vi "Experiment 21.vi"() -> ()   [LabVIEW 2026]
doc: "Experiment 21\nThis experiment is like Experiment 19 but uses while loops instead of for loops."
uses:
  <vilib>/AdvancedString/1D String Array to Delimited String (string).vi
  <vilib>/Analysis/baseanly.llb/Mean (DBL).vi
  <vilib>/Analysis/NI_AALBase.lvlib
panel:
  out "No. Of Iterations Executed - Loop 14":i32
  out "Output - Loop 14":dbl[](array[numeric]) format="%.3f"
  out "No. Of Iterations Executed - Loop 13":i32
  out "Output - Loop 13":dbl[](array[numeric]) format="%.3f"
  out "No. Of Iterations Executed - Loop 12":i32
  out "Output - Loop 12":dbl[](array[numeric]) format="%.3f"
  out "No. Of Iterations Executed - Loop 11":i32
  out "Output - Loop 11":dbl[](array[numeric]) format="%.3f"
  out "No. Of Iterations As Block Of Text (easy to copy into Excel)":string
  out "No. Of Iterations Executed - Loop 10":i32
  out "Output - Loop 10":dbl[](array[numeric]) format="%.3f"
  out "No. Of Iterations Executed - Loop 9":i32
  out "Output - Loop 9":dbl[](array[numeric]) format="%.3f"
  out "No. Of Iterations Executed - Loop 8":i32
  out "Output - Loop 8":dbl[](array[numeric]) format="%.3f"
  out "No. Of Iterations Executed - Loop 7":i32
  out "Output - Loop 7":dbl[](array[numeric]) format="%.3f"
  out "No. Of Iterations Executed - Loop 6":i32
  out "Output - Loop 6":dbl[](array[numeric]) format="%.3f"
  out "No. Of Iterations Executed - Loop 5":i32
  out "Output - Loop 5":dbl[](array[numeric]) format="%.3f"
  out "No. Of Iterations Executed - Loop 4":i32
  out "Output - Loop 4":dbl[](array[numeric]) format="%.3f"
  out "No. Of Iterations Executed - Loop 3":i32
  out "Output - Loop 3":dbl[](array[numeric]) format="%.3f"
  out "Avg. No. Of Iterations Executed - All Loops":dbl format="%.1f"
  out "No. Of Iterations Executed - Loop 2":i32
  out "Output - Loop 2":dbl[](array[numeric]) format="%.3f"
  out "No. Of Iterations Executed - Loop 1":i32
  out "Output - Loop 1":dbl[](array[numeric]) format="%.3f"
  out "Stop VI?":bool
  # "Experiment 21"
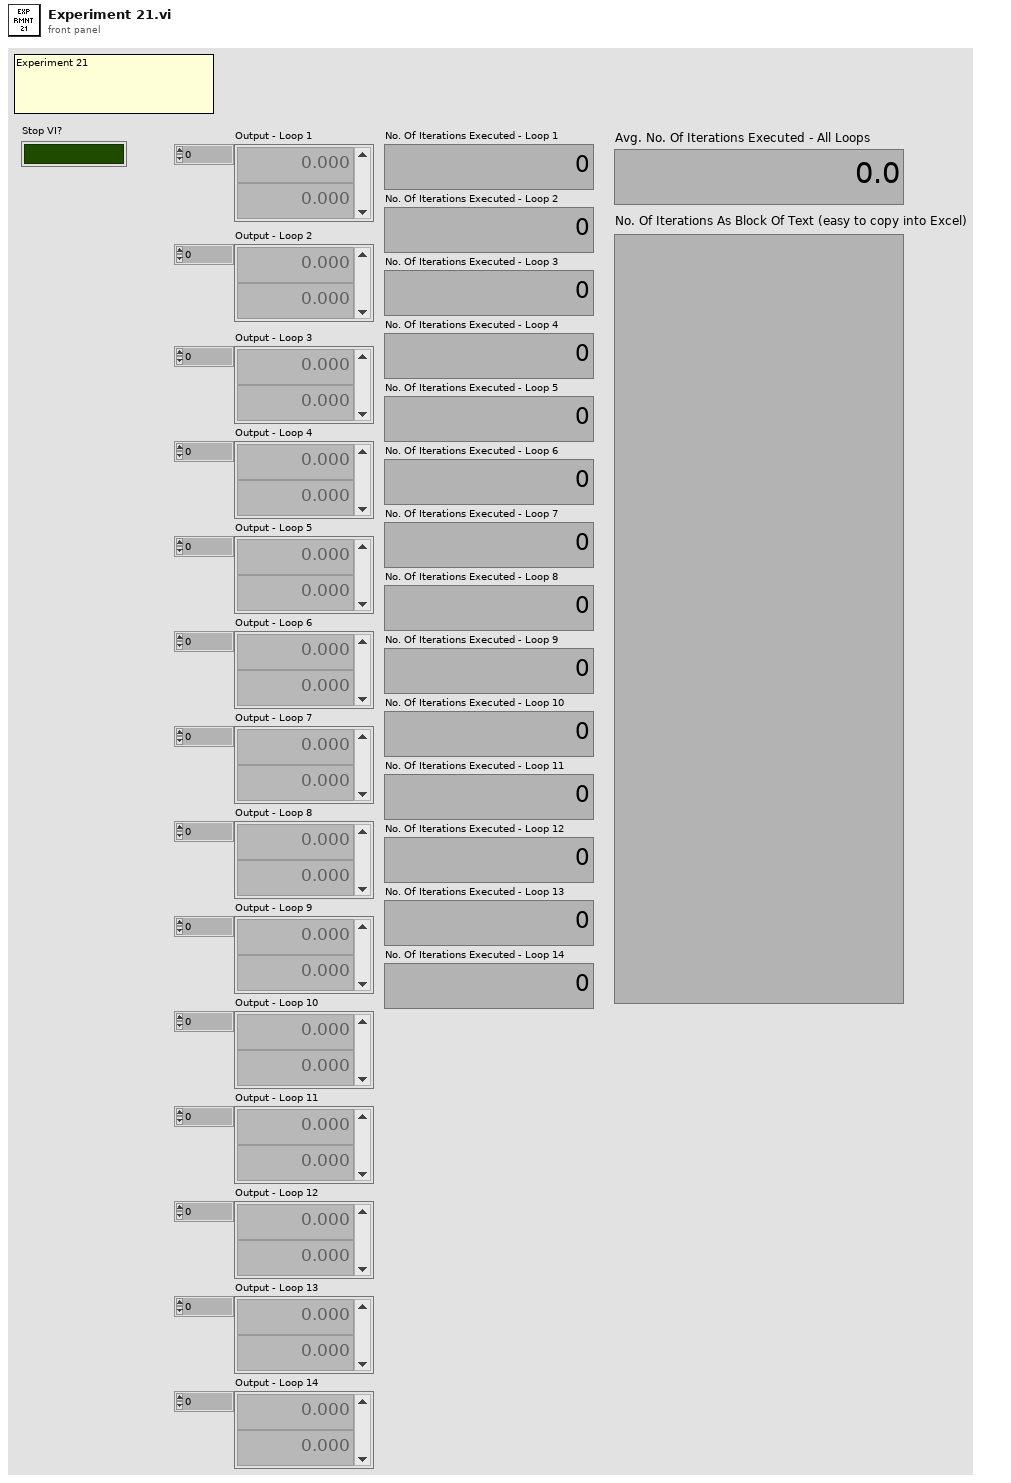
[diagram p1: front panel]
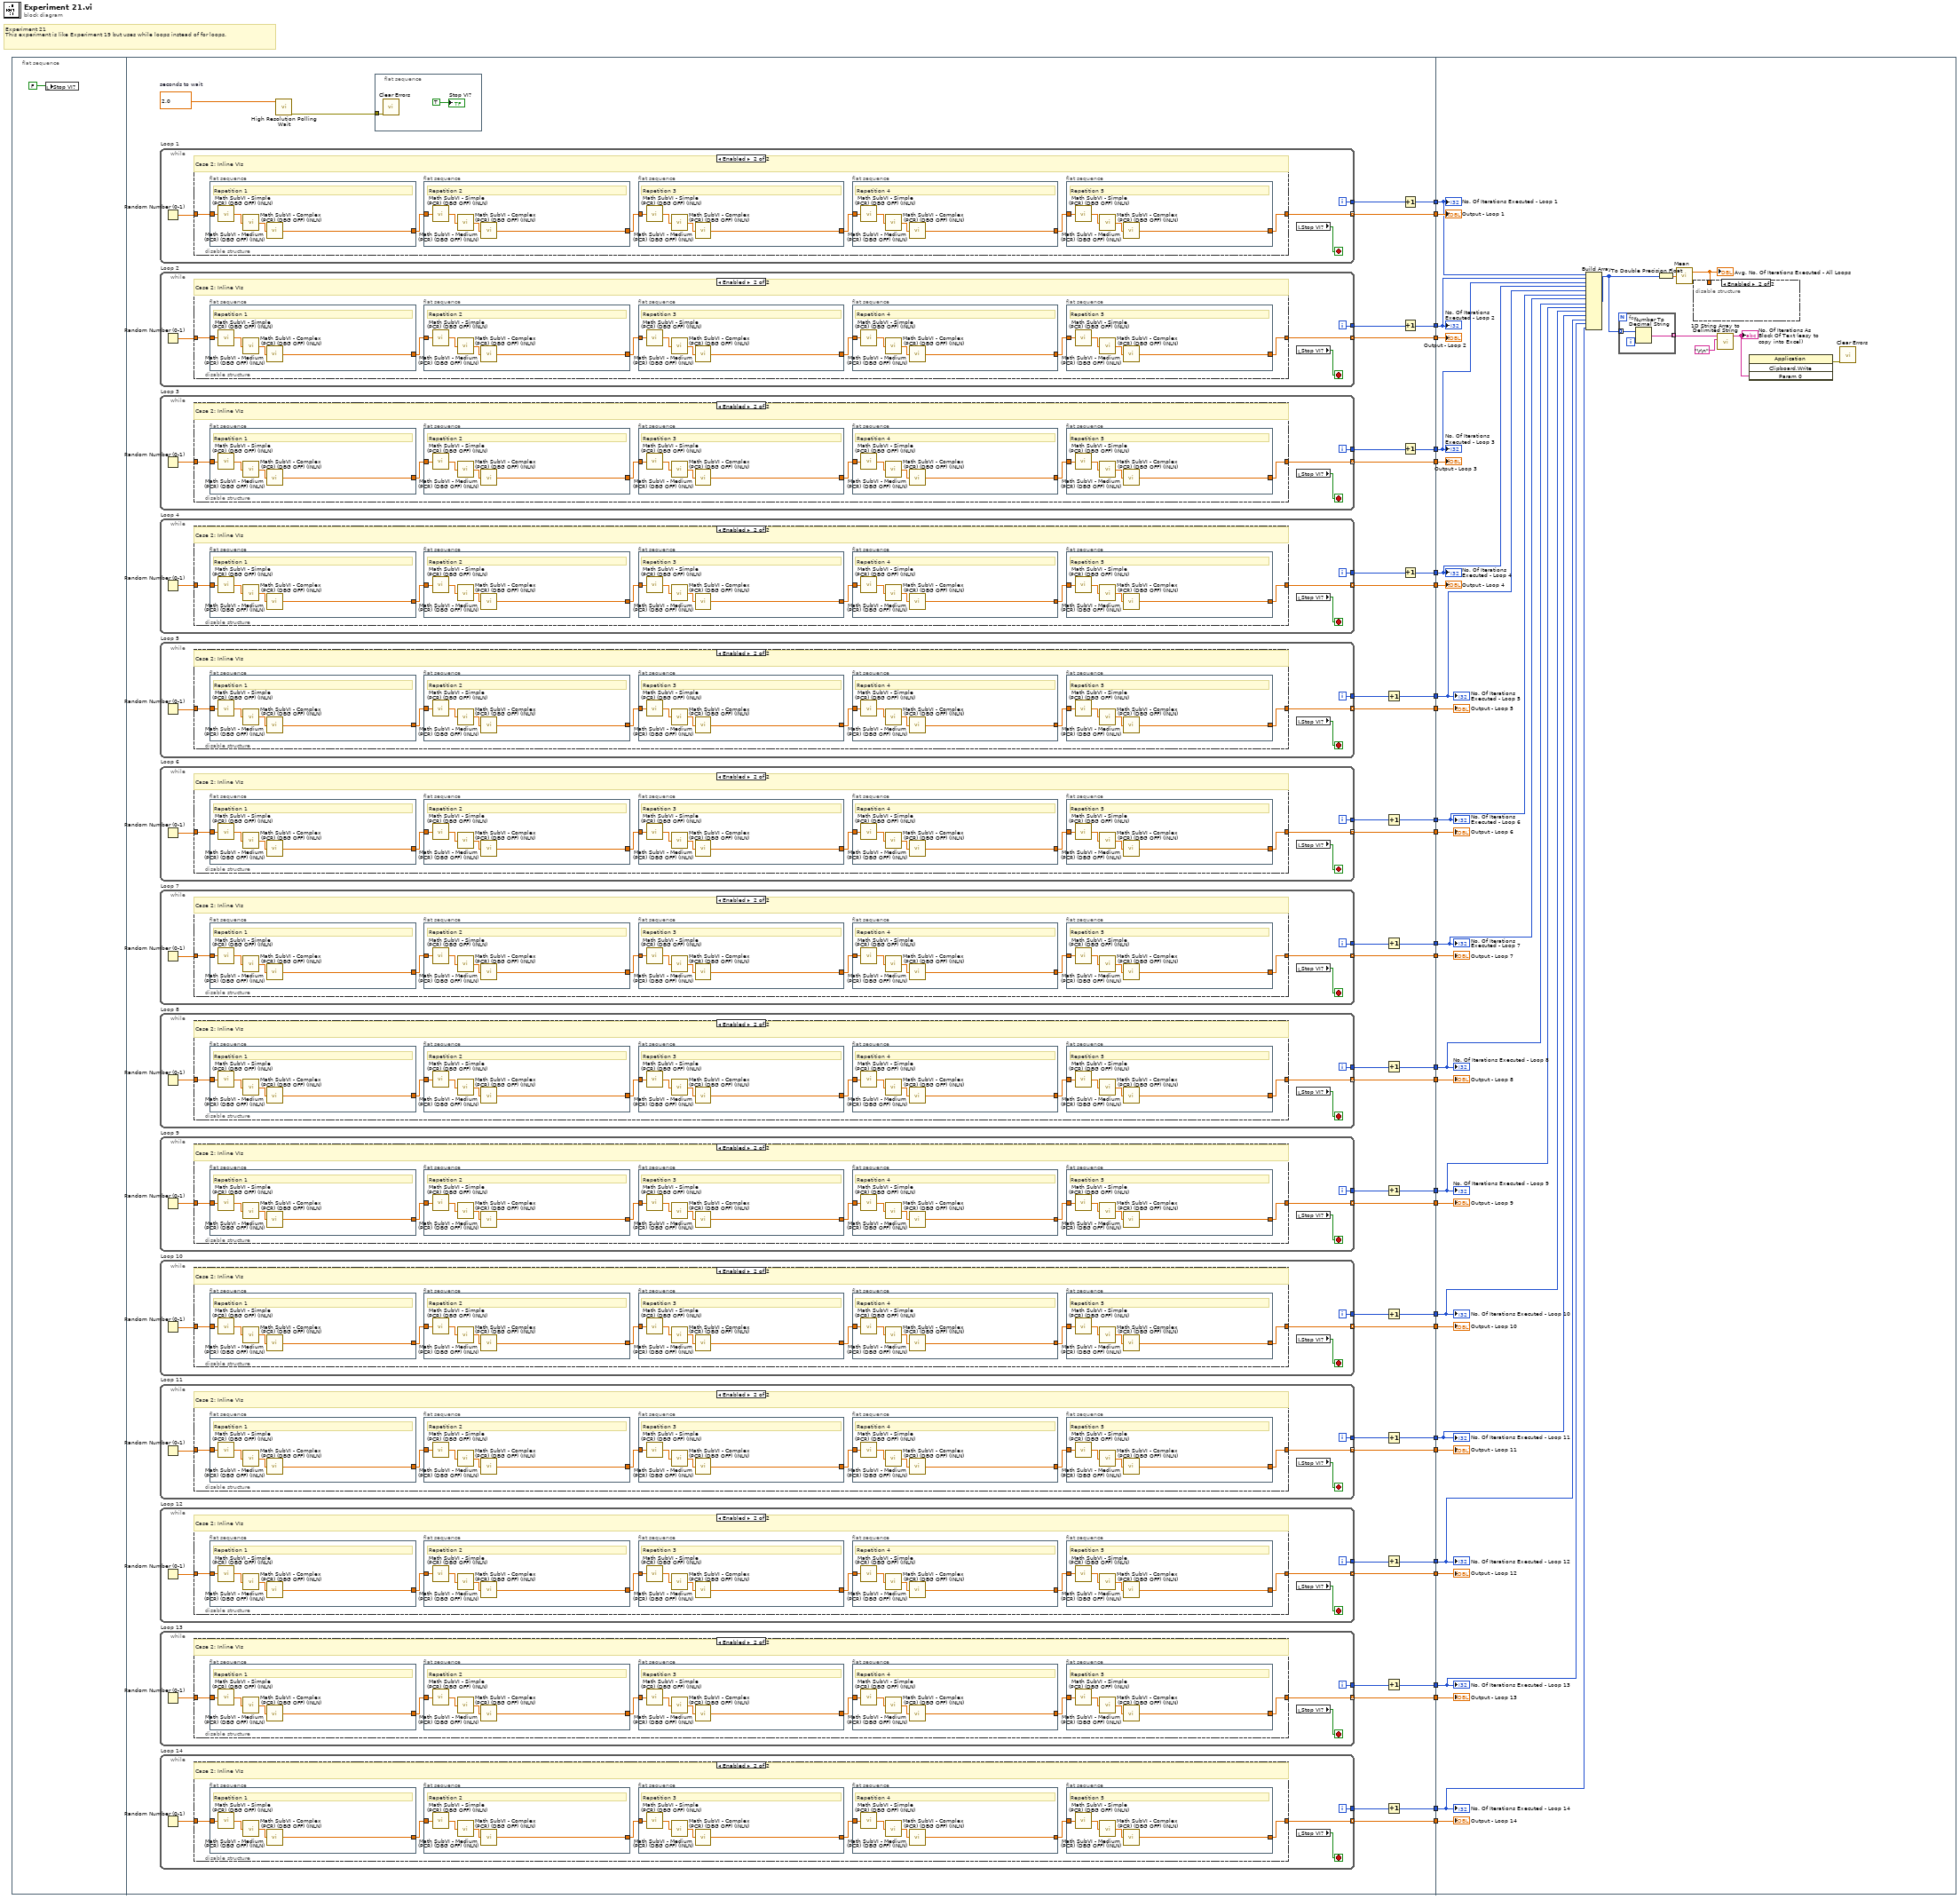
[diagram p0: block diagram]
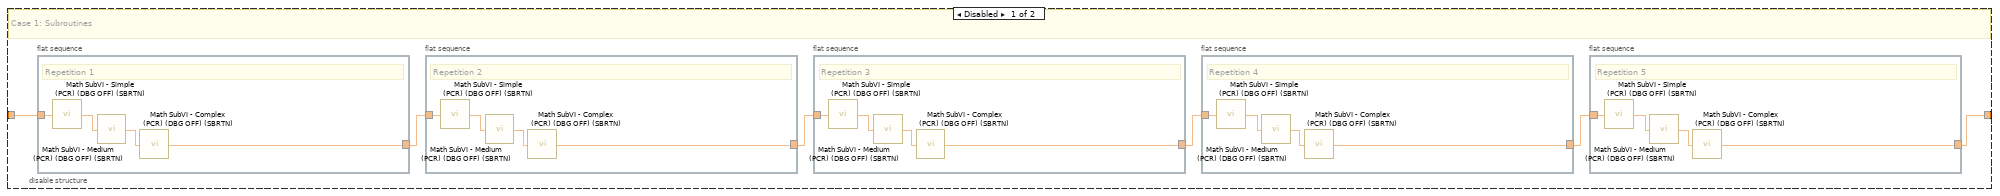
[diagram p2: hidden frame]
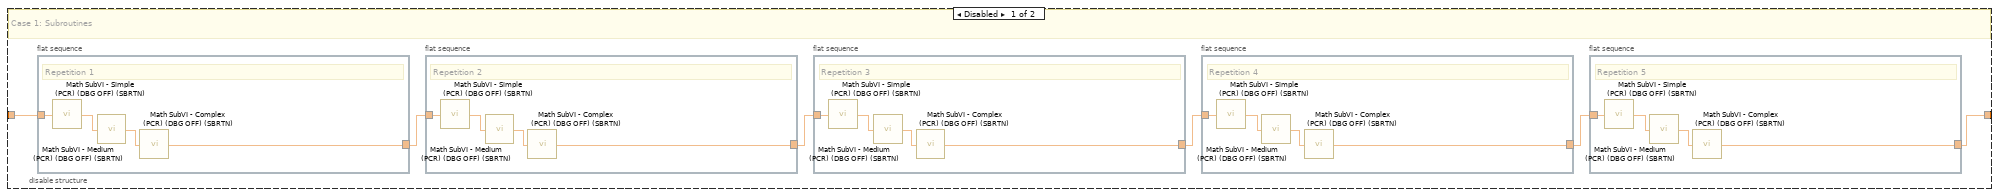
[diagram p3: hidden frame]
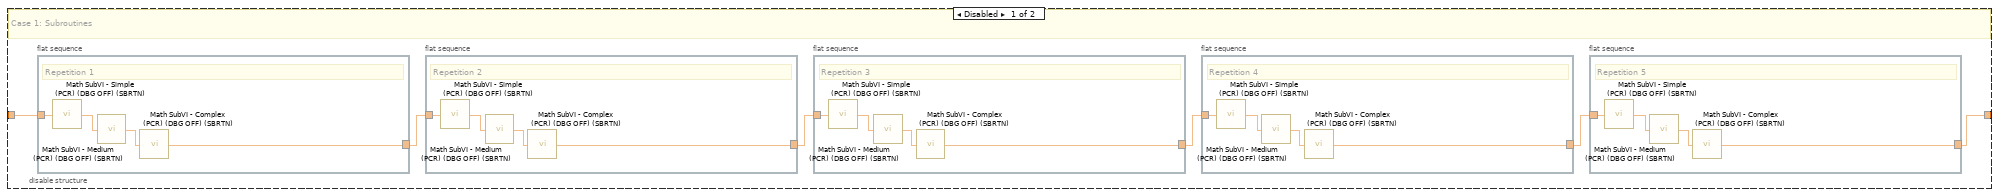
[diagram p4: hidden frame]
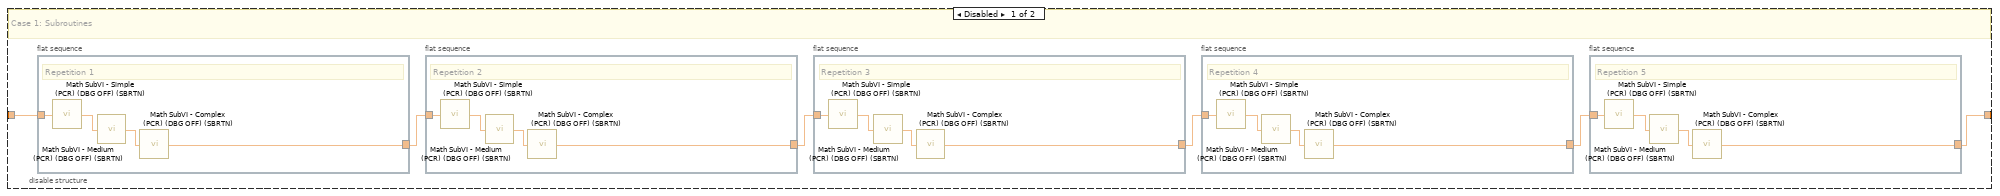
[diagram p5: hidden frame]
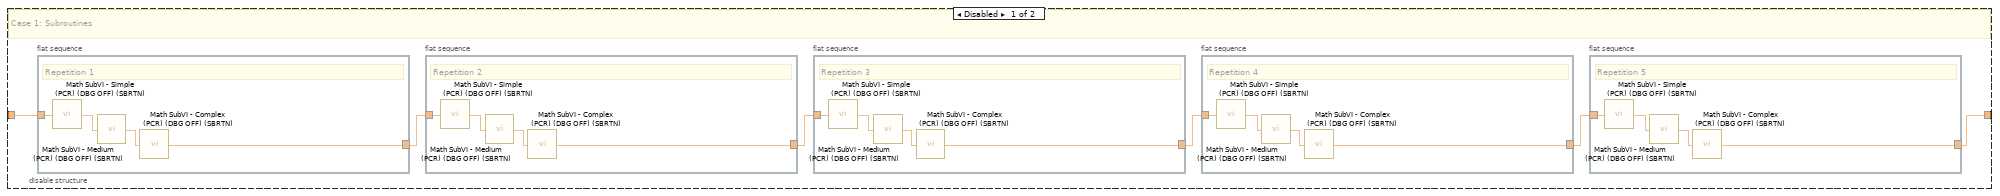
[diagram p6: hidden frame]
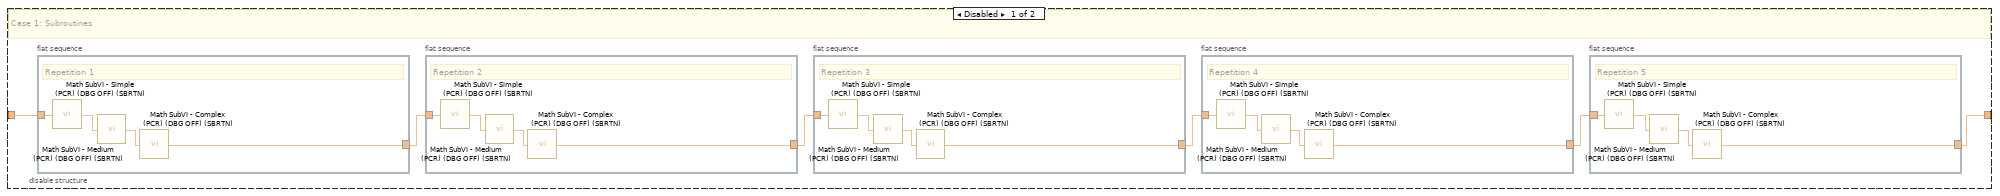
[diagram p7: hidden frame]
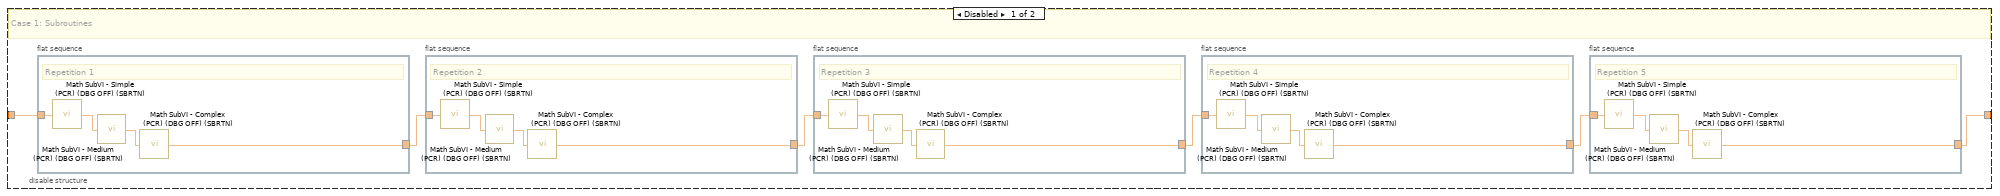
[diagram p8: hidden frame]
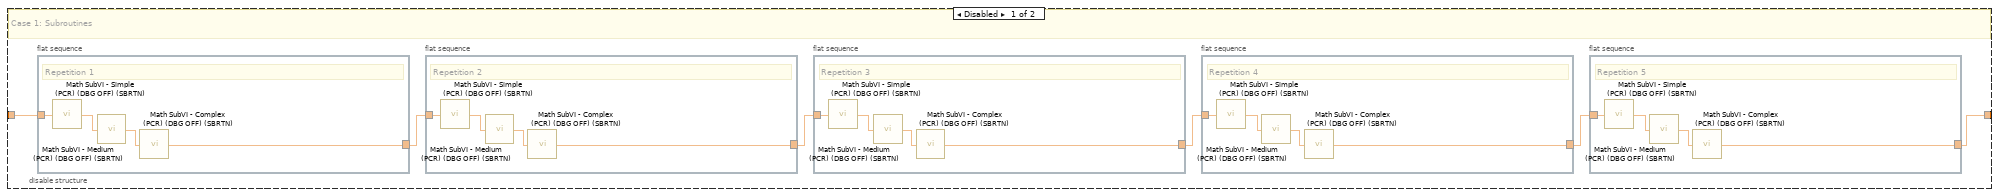
[diagram p9: hidden frame]
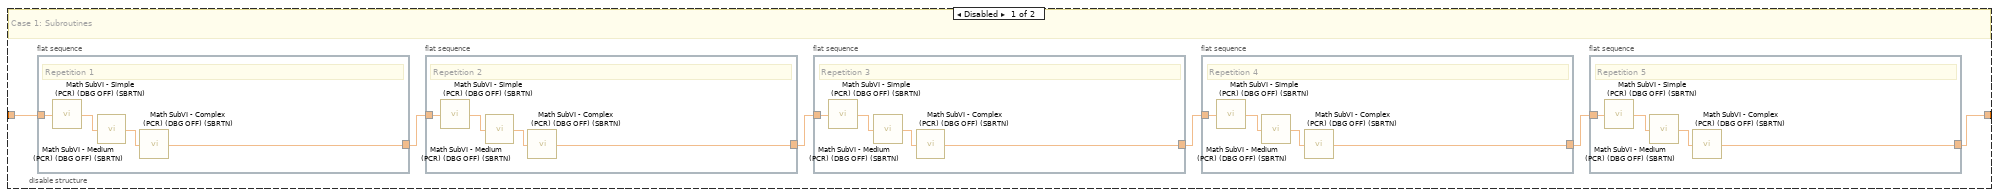
[diagram p10: hidden frame]
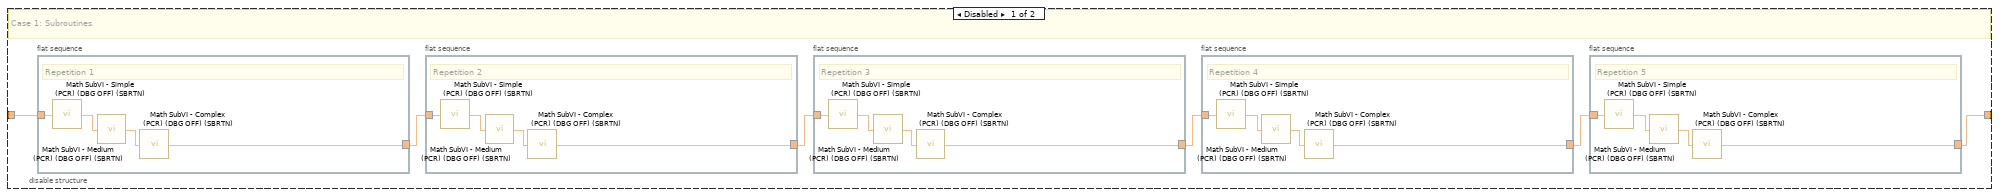
[diagram p11: hidden frame]
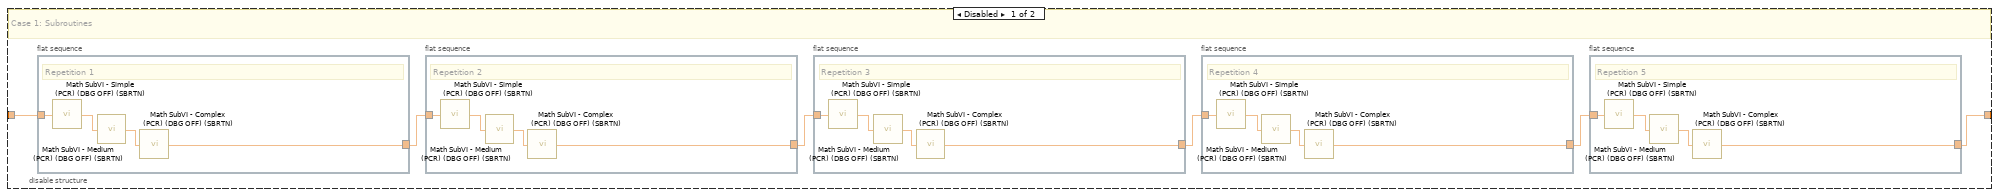
[diagram p12: hidden frame]
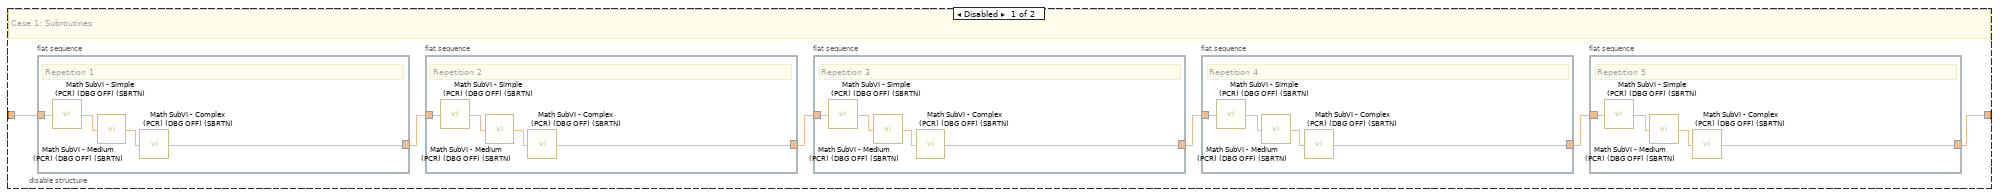
[diagram p13: hidden frame]
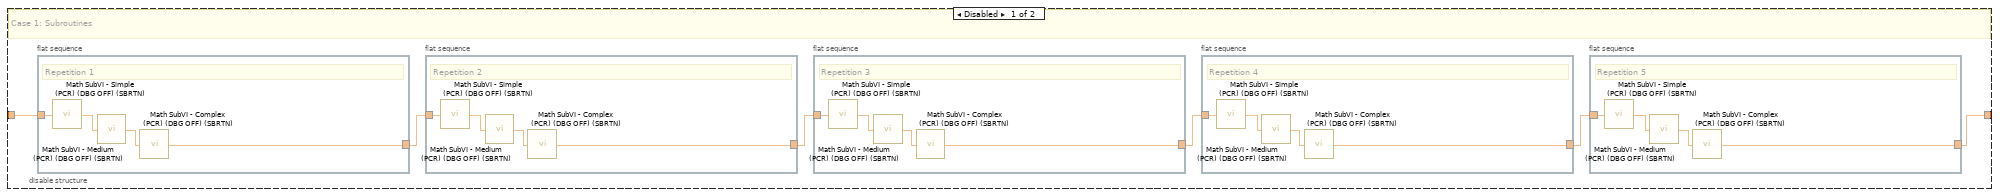
[diagram p14: hidden frame]
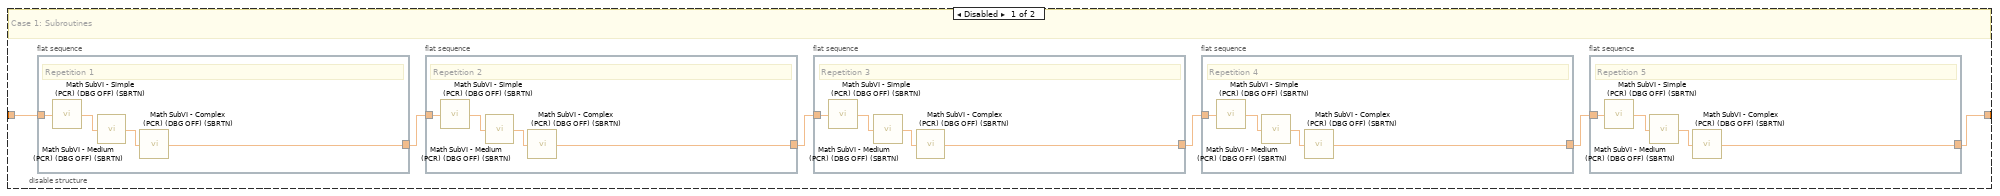
[diagram p15: hidden frame]
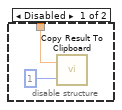
[diagram p16: hidden frame]
diagram:
  # "Experiment 21\nThis experiment is like Experiment 19 but uses while loops instead of for loops."
  n1 = flat-sequence {
    tunnel: [w71] -> w28
    tunnel: [w69] -> w27
    tunnel: [w68] -> w26
    tunnel: [w59] -> w25
    tunnel: [w67] -> w24
    tunnel: [w57] -> w23
    tunnel: [w55] -> w22
    tunnel: [w66] -> w21
    tunnel: [w53] -> w20
    tunnel: [w65] -> w19
    tunnel: [w51] -> w18
    tunnel: [w60] -> w17
    tunnel: [w49] -> w16
    tunnel: [w61] -> w15
    tunnel: [w46] -> w14
    tunnel: [w62] -> w13
    tunnel: [w44] -> w12
    tunnel: [w63] -> w11
    tunnel: [w42] -> w10
    tunnel: [w64] -> w9
    tunnel: [w41] -> w8
    tunnel: [w39] -> w7
    tunnel: [w38] -> w6
    tunnel: [w32] -> w5
    tunnel: [w36] -> w4
    tunnel: [w31] -> w3
    tunnel: [w34] -> w2
    tunnel: [w30] -> w1
    tunnel: w28 -> [w894]
    tunnel: w27 -> [w892]
    tunnel: w26 -> [w891]
    tunnel: w25 -> [w893]
    tunnel: w24 -> [w887]
    tunnel: w23 -> [w889]
    tunnel: w22 -> [w888]
    tunnel: w21 -> [w886]
    tunnel: w20 -> [w884]
    tunnel: w19 -> [w878]
    tunnel: w18 -> [w883]
    tunnel: w17 -> [w877]
    tunnel: w16 -> [w882]
    tunnel: w15 -> [w876]
    tunnel: w14 -> [w881]
    tunnel: w13 -> [w875]
    tunnel: w12 -> [w880]
    tunnel: w11 -> [w874]
    tunnel: w10 -> [w879]
    tunnel: w9 -> [w873]
    tunnel: w8 -> [w867]
    tunnel: w7 -> [w863]
    tunnel: w6 -> [w866]
    tunnel: w5 -> [w862]
    tunnel: w4 -> [w865]
    tunnel: w3 -> [w861]
    tunnel: w2 -> [w864]
    tunnel: w1 -> [w860]
    frame #0 {
      n2 = local write "Stop VI?"(FALSE) -> ()
    }
    frame #1 {
      w73 = 2.0  # seconds to wait
      n3 = while "Loop 1" {
        tunnel: [w803] -> w71 mode=indexing
        tunnel: [w804] -> w70
        i -> [w804]
        stop <- w805 stop-if-true
        n4 = Random Number (0-1)() -> (number: 0 to 1=w802:dbl)
        n5 = disable-structure shown="Enabled" {
          disable-tunnel: w802 -> [w811 w837]
          disable-tunnel: [w810 w832] -> w803
          frame Disabled {
            # "Case 1: Subroutines"
            n6 = flat-sequence {
              tunnel: w811 -> [w831]
              tunnel: [w828] -> w806
              frame #0 {
                # "Repetition 1"
                n7 = call "Math SubVI - Simple (PCR) (DBG OFF) (SBRTN).vi"("Input"=w831) -> ("Output"=w829:dbl)
                n8 = call "Math SubVI - Medium (PCR) (DBG OFF) (SBRTN).vi"("Input"=w829) -> ("Output"=w830:dbl)
                n9 = call "Math SubVI - Complex (PCR) (DBG OFF) (SBRTN).vi"("Input"=w830) -> ("Output"=w828:dbl)
              }
            }
            n10 = flat-sequence {
              tunnel: w806 -> [w827]
              tunnel: [w824] -> w809
              frame #0 {
                # "Repetition 2"
                n11 = call "Math SubVI - Simple (PCR) (DBG OFF) (SBRTN).vi"("Input"=w827) -> ("Output"=w825:dbl)
                n12 = call "Math SubVI - Medium (PCR) (DBG OFF) (SBRTN).vi"("Input"=w825) -> ("Output"=w826:dbl)
                n13 = call "Math SubVI - Complex (PCR) (DBG OFF) (SBRTN).vi"("Input"=w826) -> ("Output"=w824:dbl)
              }
            }
            n14 = flat-sequence {
              tunnel: w809 -> [w823]
              tunnel: [w820] -> w808
              frame #0 {
                # "Repetition 3"
                n15 = call "Math SubVI - Simple (PCR) (DBG OFF) (SBRTN).vi"("Input"=w823) -> ("Output"=w821:dbl)
                n16 = call "Math SubVI - Medium (PCR) (DBG OFF) (SBRTN).vi"("Input"=w821) -> ("Output"=w822:dbl)
                n17 = call "Math SubVI - Complex (PCR) (DBG OFF) (SBRTN).vi"("Input"=w822) -> ("Output"=w820:dbl)
              }
            }
            n18 = flat-sequence {
              tunnel: w808 -> [w819]
              tunnel: [w816] -> w807
              frame #0 {
                # "Repetition 4"
                n19 = call "Math SubVI - Simple (PCR) (DBG OFF) (SBRTN).vi"("Input"=w819) -> ("Output"=w817:dbl)
                n20 = call "Math SubVI - Medium (PCR) (DBG OFF) (SBRTN).vi"("Input"=w817) -> ("Output"=w818:dbl)
                n21 = call "Math SubVI - Complex (PCR) (DBG OFF) (SBRTN).vi"("Input"=w818) -> ("Output"=w816:dbl)
              }
            }
            n22 = flat-sequence {
              tunnel: w807 -> [w815]
              tunnel: [w812] -> w810
              frame #0 {
                # "Repetition 5"
                n23 = call "Math SubVI - Simple (PCR) (DBG OFF) (SBRTN).vi"("Input"=w815) -> ("Output"=w813:dbl)
                n24 = call "Math SubVI - Medium (PCR) (DBG OFF) (SBRTN).vi"("Input"=w813) -> ("Output"=w814:dbl)
                n25 = call "Math SubVI - Complex (PCR) (DBG OFF) (SBRTN).vi"("Input"=w814) -> ("Output"=w812:dbl)
              }
            }
          }
          frame Enabled {
            # "Case 2: Inline VIs"
            n26 = flat-sequence {
              tunnel: w837 -> [w857]
              tunnel: [w854] -> w836
              frame #0 {
                # "Repetition 1"
                n27 = call "Math SubVI - Simple (PCR) (DBG OFF) (INLN).vi"("Input"=w857) -> ("Output"=w855:dbl)
                n28 = call "Math SubVI - Medium (PCR) (DBG OFF) (INLN).vi"("Input"=w855) -> ("Output"=w856:dbl)
                n29 = call "Math SubVI - Complex (PCR) (DBG OFF) (INLN).vi"("Input"=w856) -> ("Output"=w854:dbl)
              }
            }
            n30 = flat-sequence {
              tunnel: w836 -> [w853]
              tunnel: [w850] -> w835
              frame #0 {
                # "Repetition 2"
                n31 = call "Math SubVI - Simple (PCR) (DBG OFF) (INLN).vi"("Input"=w853) -> ("Output"=w851:dbl)
                n32 = call "Math SubVI - Medium (PCR) (DBG OFF) (INLN).vi"("Input"=w851) -> ("Output"=w852:dbl)
                n33 = call "Math SubVI - Complex (PCR) (DBG OFF) (INLN).vi"("Input"=w852) -> ("Output"=w850:dbl)
              }
            }
            n34 = flat-sequence {
              tunnel: w835 -> [w849]
              tunnel: [w846] -> w834
              frame #0 {
                # "Repetition 3"
                n35 = call "Math SubVI - Simple (PCR) (DBG OFF) (INLN).vi"("Input"=w849) -> ("Output"=w847:dbl)
                n36 = call "Math SubVI - Medium (PCR) (DBG OFF) (INLN).vi"("Input"=w847) -> ("Output"=w848:dbl)
                n37 = call "Math SubVI - Complex (PCR) (DBG OFF) (INLN).vi"("Input"=w848) -> ("Output"=w846:dbl)
              }
            }
            n38 = flat-sequence {
              tunnel: w834 -> [w845]
              tunnel: [w842] -> w833
              frame #0 {
                # "Repetition 4"
                n39 = call "Math SubVI - Simple (PCR) (DBG OFF) (INLN).vi"("Input"=w845) -> ("Output"=w843:dbl)
                n40 = call "Math SubVI - Medium (PCR) (DBG OFF) (INLN).vi"("Input"=w843) -> ("Output"=w844:dbl)
                n41 = call "Math SubVI - Complex (PCR) (DBG OFF) (INLN).vi"("Input"=w844) -> ("Output"=w842:dbl)
              }
            }
            n42 = flat-sequence {
              tunnel: w833 -> [w841]
              tunnel: [w838] -> w832
              frame #0 {
                # "Repetition 5"
                n43 = call "Math SubVI - Simple (PCR) (DBG OFF) (INLN).vi"("Input"=w841) -> ("Output"=w839:dbl)
                n44 = call "Math SubVI - Medium (PCR) (DBG OFF) (INLN).vi"("Input"=w839) -> ("Output"=w840:dbl)
                n45 = call "Math SubVI - Complex (PCR) (DBG OFF) (INLN).vi"("Input"=w840) -> ("Output"=w838:dbl)
              }
            }
          }
        }
        n46 = local read "Stop VI?"() -> (w805:bool)
      }
      n47 = while "Loop 2" {
        tunnel: [w747] -> w59 mode=indexing
        tunnel: [w748] -> w58
        i -> [w748]
        stop <- w749 stop-if-true
        n48 = Random Number (0-1)() -> (number: 0 to 1=w746:dbl)
        n49 = disable-structure shown="Enabled" {
          disable-tunnel: w746 -> [w755 w781]
          disable-tunnel: [w754 w776] -> w747
          frame Disabled {
            # "Case 1: Subroutines"
            n50 = flat-sequence {
              tunnel: w755 -> [w775]
              tunnel: [w772] -> w750
              frame #0 {
                # "Repetition 1"
                n51 = call "Math SubVI - Simple (PCR) (DBG OFF) (SBRTN).vi"("Input"=w775) -> ("Output"=w773:dbl)
                n52 = call "Math SubVI - Medium (PCR) (DBG OFF) (SBRTN).vi"("Input"=w773) -> ("Output"=w774:dbl)
                n53 = call "Math SubVI - Complex (PCR) (DBG OFF) (SBRTN).vi"("Input"=w774) -> ("Output"=w772:dbl)
              }
            }
            n54 = flat-sequence {
              tunnel: w750 -> [w771]
              tunnel: [w768] -> w753
              frame #0 {
                # "Repetition 2"
                n55 = call "Math SubVI - Simple (PCR) (DBG OFF) (SBRTN).vi"("Input"=w771) -> ("Output"=w769:dbl)
                n56 = call "Math SubVI - Medium (PCR) (DBG OFF) (SBRTN).vi"("Input"=w769) -> ("Output"=w770:dbl)
                n57 = call "Math SubVI - Complex (PCR) (DBG OFF) (SBRTN).vi"("Input"=w770) -> ("Output"=w768:dbl)
              }
            }
            n58 = flat-sequence {
              tunnel: w753 -> [w767]
              tunnel: [w764] -> w752
              frame #0 {
                # "Repetition 3"
                n59 = call "Math SubVI - Simple (PCR) (DBG OFF) (SBRTN).vi"("Input"=w767) -> ("Output"=w765:dbl)
                n60 = call "Math SubVI - Medium (PCR) (DBG OFF) (SBRTN).vi"("Input"=w765) -> ("Output"=w766:dbl)
                n61 = call "Math SubVI - Complex (PCR) (DBG OFF) (SBRTN).vi"("Input"=w766) -> ("Output"=w764:dbl)
              }
            }
            n62 = flat-sequence {
              tunnel: w752 -> [w763]
              tunnel: [w760] -> w751
              frame #0 {
                # "Repetition 4"
                n63 = call "Math SubVI - Simple (PCR) (DBG OFF) (SBRTN).vi"("Input"=w763) -> ("Output"=w761:dbl)
                n64 = call "Math SubVI - Medium (PCR) (DBG OFF) (SBRTN).vi"("Input"=w761) -> ("Output"=w762:dbl)
                n65 = call "Math SubVI - Complex (PCR) (DBG OFF) (SBRTN).vi"("Input"=w762) -> ("Output"=w760:dbl)
              }
            }
            n66 = flat-sequence {
              tunnel: w751 -> [w759]
              tunnel: [w756] -> w754
              frame #0 {
                # "Repetition 5"
                n67 = call "Math SubVI - Simple (PCR) (DBG OFF) (SBRTN).vi"("Input"=w759) -> ("Output"=w757:dbl)
                n68 = call "Math SubVI - Medium (PCR) (DBG OFF) (SBRTN).vi"("Input"=w757) -> ("Output"=w758:dbl)
                n69 = call "Math SubVI - Complex (PCR) (DBG OFF) (SBRTN).vi"("Input"=w758) -> ("Output"=w756:dbl)
              }
            }
          }
          frame Enabled {
            # "Case 2: Inline VIs"
            n70 = flat-sequence {
              tunnel: w781 -> [w801]
              tunnel: [w798] -> w780
              frame #0 {
                # "Repetition 1"
                n71 = call "Math SubVI - Simple (PCR) (DBG OFF) (INLN).vi"("Input"=w801) -> ("Output"=w799:dbl)
                n72 = call "Math SubVI - Medium (PCR) (DBG OFF) (INLN).vi"("Input"=w799) -> ("Output"=w800:dbl)
                n73 = call "Math SubVI - Complex (PCR) (DBG OFF) (INLN).vi"("Input"=w800) -> ("Output"=w798:dbl)
              }
            }
            n74 = flat-sequence {
              tunnel: w780 -> [w797]
              tunnel: [w794] -> w779
              frame #0 {
                # "Repetition 2"
                n75 = call "Math SubVI - Simple (PCR) (DBG OFF) (INLN).vi"("Input"=w797) -> ("Output"=w795:dbl)
                n76 = call "Math SubVI - Medium (PCR) (DBG OFF) (INLN).vi"("Input"=w795) -> ("Output"=w796:dbl)
                n77 = call "Math SubVI - Complex (PCR) (DBG OFF) (INLN).vi"("Input"=w796) -> ("Output"=w794:dbl)
              }
            }
            n78 = flat-sequence {
              tunnel: w779 -> [w793]
              tunnel: [w790] -> w778
              frame #0 {
                # "Repetition 3"
                n79 = call "Math SubVI - Simple (PCR) (DBG OFF) (INLN).vi"("Input"=w793) -> ("Output"=w791:dbl)
                n80 = call "Math SubVI - Medium (PCR) (DBG OFF) (INLN).vi"("Input"=w791) -> ("Output"=w792:dbl)
                n81 = call "Math SubVI - Complex (PCR) (DBG OFF) (INLN).vi"("Input"=w792) -> ("Output"=w790:dbl)
              }
            }
            n82 = flat-sequence {
              tunnel: w778 -> [w789]
              tunnel: [w786] -> w777
              frame #0 {
                # "Repetition 4"
                n83 = call "Math SubVI - Simple (PCR) (DBG OFF) (INLN).vi"("Input"=w789) -> ("Output"=w787:dbl)
                n84 = call "Math SubVI - Medium (PCR) (DBG OFF) (INLN).vi"("Input"=w787) -> ("Output"=w788:dbl)
                n85 = call "Math SubVI - Complex (PCR) (DBG OFF) (INLN).vi"("Input"=w788) -> ("Output"=w786:dbl)
              }
            }
            n86 = flat-sequence {
              tunnel: w777 -> [w785]
              tunnel: [w782] -> w776
              frame #0 {
                # "Repetition 5"
                n87 = call "Math SubVI - Simple (PCR) (DBG OFF) (INLN).vi"("Input"=w785) -> ("Output"=w783:dbl)
                n88 = call "Math SubVI - Medium (PCR) (DBG OFF) (INLN).vi"("Input"=w783) -> ("Output"=w784:dbl)
                n89 = call "Math SubVI - Complex (PCR) (DBG OFF) (INLN).vi"("Input"=w784) -> ("Output"=w782:dbl)
              }
            }
          }
        }
        n90 = local read "Stop VI?"() -> (w749:bool)
      }
      n91 = while "Loop 3" {
        tunnel: [w691] -> w57 mode=indexing
        tunnel: [w692] -> w56
        i -> [w692]
        stop <- w693 stop-if-true
        n92 = Random Number (0-1)() -> (number: 0 to 1=w690:dbl)
        n93 = disable-structure shown="Enabled" {
          disable-tunnel: w690 -> [w699 w725]
          disable-tunnel: [w698 w720] -> w691
          frame Disabled {
            # "Case 1: Subroutines"
            n94 = flat-sequence {
              tunnel: w699 -> [w719]
              tunnel: [w716] -> w694
              frame #0 {
                # "Repetition 1"
                n95 = call "Math SubVI - Simple (PCR) (DBG OFF) (SBRTN).vi"("Input"=w719) -> ("Output"=w717:dbl)
                n96 = call "Math SubVI - Medium (PCR) (DBG OFF) (SBRTN).vi"("Input"=w717) -> ("Output"=w718:dbl)
                n97 = call "Math SubVI - Complex (PCR) (DBG OFF) (SBRTN).vi"("Input"=w718) -> ("Output"=w716:dbl)
              }
            }
            n98 = flat-sequence {
              tunnel: w694 -> [w715]
              tunnel: [w712] -> w697
              frame #0 {
                # "Repetition 2"
                n99 = call "Math SubVI - Simple (PCR) (DBG OFF) (SBRTN).vi"("Input"=w715) -> ("Output"=w713:dbl)
                n100 = call "Math SubVI - Medium (PCR) (DBG OFF) (SBRTN).vi"("Input"=w713) -> ("Output"=w714:dbl)
                n101 = call "Math SubVI - Complex (PCR) (DBG OFF) (SBRTN).vi"("Input"=w714) -> ("Output"=w712:dbl)
              }
            }
            n102 = flat-sequence {
              tunnel: w697 -> [w711]
              tunnel: [w708] -> w696
              frame #0 {
                # "Repetition 3"
                n103 = call "Math SubVI - Simple (PCR) (DBG OFF) (SBRTN).vi"("Input"=w711) -> ("Output"=w709:dbl)
                n104 = call "Math SubVI - Medium (PCR) (DBG OFF) (SBRTN).vi"("Input"=w709) -> ("Output"=w710:dbl)
                n105 = call "Math SubVI - Complex (PCR) (DBG OFF) (SBRTN).vi"("Input"=w710) -> ("Output"=w708:dbl)
              }
            }
            n106 = flat-sequence {
              tunnel: w696 -> [w707]
              tunnel: [w704] -> w695
              frame #0 {
                # "Repetition 4"
                n107 = call "Math SubVI - Simple (PCR) (DBG OFF) (SBRTN).vi"("Input"=w707) -> ("Output"=w705:dbl)
                n108 = call "Math SubVI - Medium (PCR) (DBG OFF) (SBRTN).vi"("Input"=w705) -> ("Output"=w706:dbl)
                n109 = call "Math SubVI - Complex (PCR) (DBG OFF) (SBRTN).vi"("Input"=w706) -> ("Output"=w704:dbl)
              }
            }
            n110 = flat-sequence {
              tunnel: w695 -> [w703]
              tunnel: [w700] -> w698
              frame #0 {
                # "Repetition 5"
                n111 = call "Math SubVI - Simple (PCR) (DBG OFF) (SBRTN).vi"("Input"=w703) -> ("Output"=w701:dbl)
                n112 = call "Math SubVI - Medium (PCR) (DBG OFF) (SBRTN).vi"("Input"=w701) -> ("Output"=w702:dbl)
                n113 = call "Math SubVI - Complex (PCR) (DBG OFF) (SBRTN).vi"("Input"=w702) -> ("Output"=w700:dbl)
              }
            }
          }
          frame Enabled {
            # "Case 2: Inline VIs"
            n114 = flat-sequence {
              tunnel: w725 -> [w745]
              tunnel: [w742] -> w724
              frame #0 {
                # "Repetition 1"
                n115 = call "Math SubVI - Simple (PCR) (DBG OFF) (INLN).vi"("Input"=w745) -> ("Output"=w743:dbl)
                n116 = call "Math SubVI - Medium (PCR) (DBG OFF) (INLN).vi"("Input"=w743) -> ("Output"=w744:dbl)
                n117 = call "Math SubVI - Complex (PCR) (DBG OFF) (INLN).vi"("Input"=w744) -> ("Output"=w742:dbl)
              }
            }
            n118 = flat-sequence {
              tunnel: w724 -> [w741]
              tunnel: [w738] -> w723
              frame #0 {
                # "Repetition 2"
                n119 = call "Math SubVI - Simple (PCR) (DBG OFF) (INLN).vi"("Input"=w741) -> ("Output"=w739:dbl)
                n120 = call "Math SubVI - Medium (PCR) (DBG OFF) (INLN).vi"("Input"=w739) -> ("Output"=w740:dbl)
                n121 = call "Math SubVI - Complex (PCR) (DBG OFF) (INLN).vi"("Input"=w740) -> ("Output"=w738:dbl)
              }
            }
            n122 = flat-sequence {
              tunnel: w723 -> [w737]
              tunnel: [w734] -> w722
              frame #0 {
                # "Repetition 3"
                n123 = call "Math SubVI - Simple (PCR) (DBG OFF) (INLN).vi"("Input"=w737) -> ("Output"=w735:dbl)
                n124 = call "Math SubVI - Medium (PCR) (DBG OFF) (INLN).vi"("Input"=w735) -> ("Output"=w736:dbl)
                n125 = call "Math SubVI - Complex (PCR) (DBG OFF) (INLN).vi"("Input"=w736) -> ("Output"=w734:dbl)
              }
            }
            n126 = flat-sequence {
              tunnel: w722 -> [w733]
              tunnel: [w730] -> w721
              frame #0 {
                # "Repetition 4"
                n127 = call "Math SubVI - Simple (PCR) (DBG OFF) (INLN).vi"("Input"=w733) -> ("Output"=w731:dbl)
                n128 = call "Math SubVI - Medium (PCR) (DBG OFF) (INLN).vi"("Input"=w731) -> ("Output"=w732:dbl)
                n129 = call "Math SubVI - Complex (PCR) (DBG OFF) (INLN).vi"("Input"=w732) -> ("Output"=w730:dbl)
              }
            }
            n130 = flat-sequence {
              tunnel: w721 -> [w729]
              tunnel: [w726] -> w720
              frame #0 {
                # "Repetition 5"
                n131 = call "Math SubVI - Simple (PCR) (DBG OFF) (INLN).vi"("Input"=w729) -> ("Output"=w727:dbl)
                n132 = call "Math SubVI - Medium (PCR) (DBG OFF) (INLN).vi"("Input"=w727) -> ("Output"=w728:dbl)
                n133 = call "Math SubVI - Complex (PCR) (DBG OFF) (INLN).vi"("Input"=w728) -> ("Output"=w726:dbl)
              }
            }
          }
        }
        n134 = local read "Stop VI?"() -> (w693:bool)
      }
      n135 = while "Loop 4" {
        tunnel: [w635] -> w55 mode=indexing
        tunnel: [w636] -> w54
        i -> [w636]
        stop <- w637 stop-if-true
        n136 = Random Number (0-1)() -> (number: 0 to 1=w634:dbl)
        n137 = disable-structure shown="Enabled" {
          disable-tunnel: w634 -> [w643 w669]
          disable-tunnel: [w642 w664] -> w635
          frame Disabled {
            # "Case 1: Subroutines"
            n138 = flat-sequence {
              tunnel: w643 -> [w663]
              tunnel: [w660] -> w638
              frame #0 {
                # "Repetition 1"
                n139 = call "Math SubVI - Simple (PCR) (DBG OFF) (SBRTN).vi"("Input"=w663) -> ("Output"=w661:dbl)
                n140 = call "Math SubVI - Medium (PCR) (DBG OFF) (SBRTN).vi"("Input"=w661) -> ("Output"=w662:dbl)
                n141 = call "Math SubVI - Complex (PCR) (DBG OFF) (SBRTN).vi"("Input"=w662) -> ("Output"=w660:dbl)
              }
            }
            n142 = flat-sequence {
              tunnel: w638 -> [w659]
              tunnel: [w656] -> w641
              frame #0 {
                # "Repetition 2"
                n143 = call "Math SubVI - Simple (PCR) (DBG OFF) (SBRTN).vi"("Input"=w659) -> ("Output"=w657:dbl)
                n144 = call "Math SubVI - Medium (PCR) (DBG OFF) (SBRTN).vi"("Input"=w657) -> ("Output"=w658:dbl)
                n145 = call "Math SubVI - Complex (PCR) (DBG OFF) (SBRTN).vi"("Input"=w658) -> ("Output"=w656:dbl)
              }
            }
            n146 = flat-sequence {
              tunnel: w641 -> [w655]
              tunnel: [w652] -> w640
              frame #0 {
                # "Repetition 3"
                n147 = call "Math SubVI - Simple (PCR) (DBG OFF) (SBRTN).vi"("Input"=w655) -> ("Output"=w653:dbl)
                n148 = call "Math SubVI - Medium (PCR) (DBG OFF) (SBRTN).vi"("Input"=w653) -> ("Output"=w654:dbl)
                n149 = call "Math SubVI - Complex (PCR) (DBG OFF) (SBRTN).vi"("Input"=w654) -> ("Output"=w652:dbl)
              }
            }
            n150 = flat-sequence {
              tunnel: w640 -> [w651]
              tunnel: [w648] -> w639
              frame #0 {
                # "Repetition 4"
                n151 = call "Math SubVI - Simple (PCR) (DBG OFF) (SBRTN).vi"("Input"=w651) -> ("Output"=w649:dbl)
                n152 = call "Math SubVI - Medium (PCR) (DBG OFF) (SBRTN).vi"("Input"=w649) -> ("Output"=w650:dbl)
                n153 = call "Math SubVI - Complex (PCR) (DBG OFF) (SBRTN).vi"("Input"=w650) -> ("Output"=w648:dbl)
              }
            }
            n154 = flat-sequence {
              tunnel: w639 -> [w647]
              tunnel: [w644] -> w642
              frame #0 {
                # "Repetition 5"
                n155 = call "Math SubVI - Simple (PCR) (DBG OFF) (SBRTN).vi"("Input"=w647) -> ("Output"=w645:dbl)
                n156 = call "Math SubVI - Medium (PCR) (DBG OFF) (SBRTN).vi"("Input"=w645) -> ("Output"=w646:dbl)
                n157 = call "Math SubVI - Complex (PCR) (DBG OFF) (SBRTN).vi"("Input"=w646) -> ("Output"=w644:dbl)
              }
            }
          }
          frame Enabled {
            # "Case 2: Inline VIs"
            n158 = flat-sequence {
              tunnel: w669 -> [w689]
              tunnel: [w686] -> w668
              frame #0 {
                # "Repetition 1"
                n159 = call "Math SubVI - Simple (PCR) (DBG OFF) (INLN).vi"("Input"=w689) -> ("Output"=w687:dbl)
                n160 = call "Math SubVI - Medium (PCR) (DBG OFF) (INLN).vi"("Input"=w687) -> ("Output"=w688:dbl)
                n161 = call "Math SubVI - Complex (PCR) (DBG OFF) (INLN).vi"("Input"=w688) -> ("Output"=w686:dbl)
              }
            }
            n162 = flat-sequence {
              tunnel: w668 -> [w685]
              tunnel: [w682] -> w667
              frame #0 {
                # "Repetition 2"
                n163 = call "Math SubVI - Simple (PCR) (DBG OFF) (INLN).vi"("Input"=w685) -> ("Output"=w683:dbl)
                n164 = call "Math SubVI - Medium (PCR) (DBG OFF) (INLN).vi"("Input"=w683) -> ("Output"=w684:dbl)
                n165 = call "Math SubVI - Complex (PCR) (DBG OFF) (INLN).vi"("Input"=w684) -> ("Output"=w682:dbl)
              }
            }
            n166 = flat-sequence {
              tunnel: w667 -> [w681]
              tunnel: [w678] -> w666
              frame #0 {
                # "Repetition 3"
                n167 = call "Math SubVI - Simple (PCR) (DBG OFF) (INLN).vi"("Input"=w681) -> ("Output"=w679:dbl)
                n168 = call "Math SubVI - Medium (PCR) (DBG OFF) (INLN).vi"("Input"=w679) -> ("Output"=w680:dbl)
                n169 = call "Math SubVI - Complex (PCR) (DBG OFF) (INLN).vi"("Input"=w680) -> ("Output"=w678:dbl)
              }
            }
            n170 = flat-sequence {
              tunnel: w666 -> [w677]
              tunnel: [w674] -> w665
              frame #0 {
                # "Repetition 4"
                n171 = call "Math SubVI - Simple (PCR) (DBG OFF) (INLN).vi"("Input"=w677) -> ("Output"=w675:dbl)
                n172 = call "Math SubVI - Medium (PCR) (DBG OFF) (INLN).vi"("Input"=w675) -> ("Output"=w676:dbl)
                n173 = call "Math SubVI - Complex (PCR) (DBG OFF) (INLN).vi"("Input"=w676) -> ("Output"=w674:dbl)
              }
            }
            n174 = flat-sequence {
              tunnel: w665 -> [w673]
              tunnel: [w670] -> w664
              frame #0 {
                # "Repetition 5"
                n175 = call "Math SubVI - Simple (PCR) (DBG OFF) (INLN).vi"("Input"=w673) -> ("Output"=w671:dbl)
                n176 = call "Math SubVI - Medium (PCR) (DBG OFF) (INLN).vi"("Input"=w671) -> ("Output"=w672:dbl)
                n177 = call "Math SubVI - Complex (PCR) (DBG OFF) (INLN).vi"("Input"=w672) -> ("Output"=w670:dbl)
              }
            }
          }
        }
        n178 = local read "Stop VI?"() -> (w637:bool)
      }
      n179 = while "Loop 5" {
        tunnel: [w579] -> w53 mode=indexing
        tunnel: [w580] -> w52
        i -> [w580]
        stop <- w581 stop-if-true
        n180 = Random Number (0-1)() -> (number: 0 to 1=w578:dbl)
        n181 = disable-structure shown="Enabled" {
          disable-tunnel: w578 -> [w587 w613]
          disable-tunnel: [w586 w608] -> w579
          frame Disabled {
            # "Case 1: Subroutines"
            n182 = flat-sequence {
              tunnel: w587 -> [w607]
              tunnel: [w604] -> w582
              frame #0 {
                # "Repetition 1"
                n183 = call "Math SubVI - Simple (PCR) (DBG OFF) (SBRTN).vi"("Input"=w607) -> ("Output"=w605:dbl)
                n184 = call "Math SubVI - Medium (PCR) (DBG OFF) (SBRTN).vi"("Input"=w605) -> ("Output"=w606:dbl)
                n185 = call "Math SubVI - Complex (PCR) (DBG OFF) (SBRTN).vi"("Input"=w606) -> ("Output"=w604:dbl)
              }
            }
            n186 = flat-sequence {
              tunnel: w582 -> [w603]
              tunnel: [w600] -> w585
              frame #0 {
                # "Repetition 2"
                n187 = call "Math SubVI - Simple (PCR) (DBG OFF) (SBRTN).vi"("Input"=w603) -> ("Output"=w601:dbl)
                n188 = call "Math SubVI - Medium (PCR) (DBG OFF) (SBRTN).vi"("Input"=w601) -> ("Output"=w602:dbl)
                n189 = call "Math SubVI - Complex (PCR) (DBG OFF) (SBRTN).vi"("Input"=w602) -> ("Output"=w600:dbl)
              }
            }
            n190 = flat-sequence {
              tunnel: w585 -> [w599]
              tunnel: [w596] -> w584
              frame #0 {
                # "Repetition 3"
                n191 = call "Math SubVI - Simple (PCR) (DBG OFF) (SBRTN).vi"("Input"=w599) -> ("Output"=w597:dbl)
                n192 = call "Math SubVI - Medium (PCR) (DBG OFF) (SBRTN).vi"("Input"=w597) -> ("Output"=w598:dbl)
                n193 = call "Math SubVI - Complex (PCR) (DBG OFF) (SBRTN).vi"("Input"=w598) -> ("Output"=w596:dbl)
              }
            }
            n194 = flat-sequence {
              tunnel: w584 -> [w595]
              tunnel: [w592] -> w583
              frame #0 {
                # "Repetition 4"
                n195 = call "Math SubVI - Simple (PCR) (DBG OFF) (SBRTN).vi"("Input"=w595) -> ("Output"=w593:dbl)
                n196 = call "Math SubVI - Medium (PCR) (DBG OFF) (SBRTN).vi"("Input"=w593) -> ("Output"=w594:dbl)
                n197 = call "Math SubVI - Complex (PCR) (DBG OFF) (SBRTN).vi"("Input"=w594) -> ("Output"=w592:dbl)
              }
            }
            n198 = flat-sequence {
              tunnel: w583 -> [w591]
              tunnel: [w588] -> w586
              frame #0 {
                # "Repetition 5"
                n199 = call "Math SubVI - Simple (PCR) (DBG OFF) (SBRTN).vi"("Input"=w591) -> ("Output"=w589:dbl)
                n200 = call "Math SubVI - Medium (PCR) (DBG OFF) (SBRTN).vi"("Input"=w589) -> ("Output"=w590:dbl)
                n201 = call "Math SubVI - Complex (PCR) (DBG OFF) (SBRTN).vi"("Input"=w590) -> ("Output"=w588:dbl)
              }
            }
          }
          frame Enabled {
            # "Case 2: Inline VIs"
            n202 = flat-sequence {
              tunnel: w613 -> [w633]
              tunnel: [w630] -> w612
              frame #0 {
                # "Repetition 1"
                n203 = call "Math SubVI - Simple (PCR) (DBG OFF) (INLN).vi"("Input"=w633) -> ("Output"=w631:dbl)
                n204 = call "Math SubVI - Medium (PCR) (DBG OFF) (INLN).vi"("Input"=w631) -> ("Output"=w632:dbl)
                n205 = call "Math SubVI - Complex (PCR) (DBG OFF) (INLN).vi"("Input"=w632) -> ("Output"=w630:dbl)
              }
            }
            n206 = flat-sequence {
              tunnel: w612 -> [w629]
              tunnel: [w626] -> w611
              frame #0 {
                # "Repetition 2"
                n207 = call "Math SubVI - Simple (PCR) (DBG OFF) (INLN).vi"("Input"=w629) -> ("Output"=w627:dbl)
                n208 = call "Math SubVI - Medium (PCR) (DBG OFF) (INLN).vi"("Input"=w627) -> ("Output"=w628:dbl)
                n209 = call "Math SubVI - Complex (PCR) (DBG OFF) (INLN).vi"("Input"=w628) -> ("Output"=w626:dbl)
              }
            }
            n210 = flat-sequence {
              tunnel: w611 -> [w625]
              tunnel: [w622] -> w610
              frame #0 {
                # "Repetition 3"
                n211 = call "Math SubVI - Simple (PCR) (DBG OFF) (INLN).vi"("Input"=w625) -> ("Output"=w623:dbl)
                n212 = call "Math SubVI - Medium (PCR) (DBG OFF) (INLN).vi"("Input"=w623) -> ("Output"=w624:dbl)
                n213 = call "Math SubVI - Complex (PCR) (DBG OFF) (INLN).vi"("Input"=w624) -> ("Output"=w622:dbl)
              }
            }
            n214 = flat-sequence {
              tunnel: w610 -> [w621]
              tunnel: [w618] -> w609
              frame #0 {
                # "Repetition 4"
                n215 = call "Math SubVI - Simple (PCR) (DBG OFF) (INLN).vi"("Input"=w621) -> ("Output"=w619:dbl)
                n216 = call "Math SubVI - Medium (PCR) (DBG OFF) (INLN).vi"("Input"=w619) -> ("Output"=w620:dbl)
                n217 = call "Math SubVI - Complex (PCR) (DBG OFF) (INLN).vi"("Input"=w620) -> ("Output"=w618:dbl)
              }
            }
            n218 = flat-sequence {
              tunnel: w609 -> [w617]
              tunnel: [w614] -> w608
              frame #0 {
                # "Repetition 5"
                n219 = call "Math SubVI - Simple (PCR) (DBG OFF) (INLN).vi"("Input"=w617) -> ("Output"=w615:dbl)
                n220 = call "Math SubVI - Medium (PCR) (DBG OFF) (INLN).vi"("Input"=w615) -> ("Output"=w616:dbl)
                n221 = call "Math SubVI - Complex (PCR) (DBG OFF) (INLN).vi"("Input"=w616) -> ("Output"=w614:dbl)
              }
            }
          }
        }
        n222 = local read "Stop VI?"() -> (w581:bool)
      }
      n223 = while "Loop 6" {
        tunnel: [w523] -> w51 mode=indexing
        tunnel: [w524] -> w50
        i -> [w524]
        stop <- w525 stop-if-true
        n224 = Random Number (0-1)() -> (number: 0 to 1=w522:dbl)
        n225 = disable-structure shown="Enabled" {
          disable-tunnel: w522 -> [w531 w557]
          disable-tunnel: [w530 w552] -> w523
          frame Disabled {
            # "Case 1: Subroutines"
            n226 = flat-sequence {
              tunnel: w531 -> [w551]
              tunnel: [w548] -> w526
              frame #0 {
                # "Repetition 1"
                n227 = call "Math SubVI - Simple (PCR) (DBG OFF) (SBRTN).vi"("Input"=w551) -> ("Output"=w549:dbl)
                n228 = call "Math SubVI - Medium (PCR) (DBG OFF) (SBRTN).vi"("Input"=w549) -> ("Output"=w550:dbl)
                n229 = call "Math SubVI - Complex (PCR) (DBG OFF) (SBRTN).vi"("Input"=w550) -> ("Output"=w548:dbl)
              }
            }
            n230 = flat-sequence {
              tunnel: w526 -> [w547]
              tunnel: [w544] -> w529
              frame #0 {
                # "Repetition 2"
                n231 = call "Math SubVI - Simple (PCR) (DBG OFF) (SBRTN).vi"("Input"=w547) -> ("Output"=w545:dbl)
                n232 = call "Math SubVI - Medium (PCR) (DBG OFF) (SBRTN).vi"("Input"=w545) -> ("Output"=w546:dbl)
                n233 = call "Math SubVI - Complex (PCR) (DBG OFF) (SBRTN).vi"("Input"=w546) -> ("Output"=w544:dbl)
              }
            }
            n234 = flat-sequence {
              tunnel: w529 -> [w543]
              tunnel: [w540] -> w528
              frame #0 {
                # "Repetition 3"
                n235 = call "Math SubVI - Simple (PCR) (DBG OFF) (SBRTN).vi"("Input"=w543) -> ("Output"=w541:dbl)
                n236 = call "Math SubVI - Medium (PCR) (DBG OFF) (SBRTN).vi"("Input"=w541) -> ("Output"=w542:dbl)
                n237 = call "Math SubVI - Complex (PCR) (DBG OFF) (SBRTN).vi"("Input"=w542) -> ("Output"=w540:dbl)
              }
            }
            n238 = flat-sequence {
              tunnel: w528 -> [w539]
              tunnel: [w536] -> w527
              frame #0 {
                # "Repetition 4"
                n239 = call "Math SubVI - Simple (PCR) (DBG OFF) (SBRTN).vi"("Input"=w539) -> ("Output"=w537:dbl)
                n240 = call "Math SubVI - Medium (PCR) (DBG OFF) (SBRTN).vi"("Input"=w537) -> ("Output"=w538:dbl)
                n241 = call "Math SubVI - Complex (PCR) (DBG OFF) (SBRTN).vi"("Input"=w538) -> ("Output"=w536:dbl)
              }
            }
            n242 = flat-sequence {
              tunnel: w527 -> [w535]
              tunnel: [w532] -> w530
              frame #0 {
                # "Repetition 5"
                n243 = call "Math SubVI - Simple (PCR) (DBG OFF) (SBRTN).vi"("Input"=w535) -> ("Output"=w533:dbl)
                n244 = call "Math SubVI - Medium (PCR) (DBG OFF) (SBRTN).vi"("Input"=w533) -> ("Output"=w534:dbl)
                n245 = call "Math SubVI - Complex (PCR) (DBG OFF) (SBRTN).vi"("Input"=w534) -> ("Output"=w532:dbl)
              }
            }
          }
          frame Enabled {
            # "Case 2: Inline VIs"
            n246 = flat-sequence {
              tunnel: w557 -> [w577]
              tunnel: [w574] -> w556
              frame #0 {
                # "Repetition 1"
                n247 = call "Math SubVI - Simple (PCR) (DBG OFF) (INLN).vi"("Input"=w577) -> ("Output"=w575:dbl)
                n248 = call "Math SubVI - Medium (PCR) (DBG OFF) (INLN).vi"("Input"=w575) -> ("Output"=w576:dbl)
                n249 = call "Math SubVI - Complex (PCR) (DBG OFF) (INLN).vi"("Input"=w576) -> ("Output"=w574:dbl)
              }
            }
            n250 = flat-sequence {
              tunnel: w556 -> [w573]
              tunnel: [w570] -> w555
              frame #0 {
                # "Repetition 2"
                n251 = call "Math SubVI - Simple (PCR) (DBG OFF) (INLN).vi"("Input"=w573) -> ("Output"=w571:dbl)
                n252 = call "Math SubVI - Medium (PCR) (DBG OFF) (INLN).vi"("Input"=w571) -> ("Output"=w572:dbl)
                n253 = call "Math SubVI - Complex (PCR) (DBG OFF) (INLN).vi"("Input"=w572) -> ("Output"=w570:dbl)
              }
            }
            n254 = flat-sequence {
              tunnel: w555 -> [w569]
              tunnel: [w566] -> w554
              frame #0 {
                # "Repetition 3"
                n255 = call "Math SubVI - Simple (PCR) (DBG OFF) (INLN).vi"("Input"=w569) -> ("Output"=w567:dbl)
                n256 = call "Math SubVI - Medium (PCR) (DBG OFF) (INLN).vi"("Input"=w567) -> ("Output"=w568:dbl)
                n257 = call "Math SubVI - Complex (PCR) (DBG OFF) (INLN).vi"("Input"=w568) -> ("Output"=w566:dbl)
              }
            }
            n258 = flat-sequence {
              tunnel: w554 -> [w565]
              tunnel: [w562] -> w553
              frame #0 {
                # "Repetition 4"
                n259 = call "Math SubVI - Simple (PCR) (DBG OFF) (INLN).vi"("Input"=w565) -> ("Output"=w563:dbl)
                n260 = call "Math SubVI - Medium (PCR) (DBG OFF) (INLN).vi"("Input"=w563) -> ("Output"=w564:dbl)
                n261 = call "Math SubVI - Complex (PCR) (DBG OFF) (INLN).vi"("Input"=w564) -> ("Output"=w562:dbl)
              }
            }
            n262 = flat-sequence {
              tunnel: w553 -> [w561]
              tunnel: [w558] -> w552
              frame #0 {
                # "Repetition 5"
                n263 = call "Math SubVI - Simple (PCR) (DBG OFF) (INLN).vi"("Input"=w561) -> ("Output"=w559:dbl)
                n264 = call "Math SubVI - Medium (PCR) (DBG OFF) (INLN).vi"("Input"=w559) -> ("Output"=w560:dbl)
                n265 = call "Math SubVI - Complex (PCR) (DBG OFF) (INLN).vi"("Input"=w560) -> ("Output"=w558:dbl)
              }
            }
          }
        }
        n266 = local read "Stop VI?"() -> (w525:bool)
      }
      n267 = while "Loop 7" {
        tunnel: [w467] -> w49 mode=indexing
        tunnel: [w468] -> w48
        i -> [w468]
        stop <- w469 stop-if-true
        n268 = Random Number (0-1)() -> (number: 0 to 1=w466:dbl)
        n269 = disable-structure shown="Enabled" {
          disable-tunnel: w466 -> [w475 w501]
          disable-tunnel: [w474 w496] -> w467
          frame Disabled {
            # "Case 1: Subroutines"
            n270 = flat-sequence {
              tunnel: w475 -> [w495]
              tunnel: [w492] -> w470
              frame #0 {
                # "Repetition 1"
                n271 = call "Math SubVI - Simple (PCR) (DBG OFF) (SBRTN).vi"("Input"=w495) -> ("Output"=w493:dbl)
                n272 = call "Math SubVI - Medium (PCR) (DBG OFF) (SBRTN).vi"("Input"=w493) -> ("Output"=w494:dbl)
                n273 = call "Math SubVI - Complex (PCR) (DBG OFF) (SBRTN).vi"("Input"=w494) -> ("Output"=w492:dbl)
              }
            }
            n274 = flat-sequence {
              tunnel: w470 -> [w491]
              tunnel: [w488] -> w473
              frame #0 {
                # "Repetition 2"
                n275 = call "Math SubVI - Simple (PCR) (DBG OFF) (SBRTN).vi"("Input"=w491) -> ("Output"=w489:dbl)
                n276 = call "Math SubVI - Medium (PCR) (DBG OFF) (SBRTN).vi"("Input"=w489) -> ("Output"=w490:dbl)
                n277 = call "Math SubVI - Complex (PCR) (DBG OFF) (SBRTN).vi"("Input"=w490) -> ("Output"=w488:dbl)
              }
            }
            n278 = flat-sequence {
              tunnel: w473 -> [w487]
              tunnel: [w484] -> w472
              frame #0 {
                # "Repetition 3"
                n279 = call "Math SubVI - Simple (PCR) (DBG OFF) (SBRTN).vi"("Input"=w487) -> ("Output"=w485:dbl)
                n280 = call "Math SubVI - Medium (PCR) (DBG OFF) (SBRTN).vi"("Input"=w485) -> ("Output"=w486:dbl)
                n281 = call "Math SubVI - Complex (PCR) (DBG OFF) (SBRTN).vi"("Input"=w486) -> ("Output"=w484:dbl)
              }
            }
            n282 = flat-sequence {
              tunnel: w472 -> [w483]
              tunnel: [w480] -> w471
              frame #0 {
                # "Repetition 4"
                n283 = call "Math SubVI - Simple (PCR) (DBG OFF) (SBRTN).vi"("Input"=w483) -> ("Output"=w481:dbl)
                n284 = call "Math SubVI - Medium (PCR) (DBG OFF) (SBRTN).vi"("Input"=w481) -> ("Output"=w482:dbl)
                n285 = call "Math SubVI - Complex (PCR) (DBG OFF) (SBRTN).vi"("Input"=w482) -> ("Output"=w480:dbl)
              }
            }
            n286 = flat-sequence {
              tunnel: w471 -> [w479]
              tunnel: [w476] -> w474
              frame #0 {
                # "Repetition 5"
                n287 = call "Math SubVI - Simple (PCR) (DBG OFF) (SBRTN).vi"("Input"=w479) -> ("Output"=w477:dbl)
                n288 = call "Math SubVI - Medium (PCR) (DBG OFF) (SBRTN).vi"("Input"=w477) -> ("Output"=w478:dbl)
                n289 = call "Math SubVI - Complex (PCR) (DBG OFF) (SBRTN).vi"("Input"=w478) -> ("Output"=w476:dbl)
              }
            }
          }
          frame Enabled {
            # "Case 2: Inline VIs"
            n290 = flat-sequence {
              tunnel: w501 -> [w521]
              tunnel: [w518] -> w500
              frame #0 {
                # "Repetition 1"
                n291 = call "Math SubVI - Simple (PCR) (DBG OFF) (INLN).vi"("Input"=w521) -> ("Output"=w519:dbl)
                n292 = call "Math SubVI - Medium (PCR) (DBG OFF) (INLN).vi"("Input"=w519) -> ("Output"=w520:dbl)
                n293 = call "Math SubVI - Complex (PCR) (DBG OFF) (INLN).vi"("Input"=w520) -> ("Output"=w518:dbl)
              }
            }
            n294 = flat-sequence {
              tunnel: w500 -> [w517]
              tunnel: [w514] -> w499
              frame #0 {
                # "Repetition 2"
                n295 = call "Math SubVI - Simple (PCR) (DBG OFF) (INLN).vi"("Input"=w517) -> ("Output"=w515:dbl)
                n296 = call "Math SubVI - Medium (PCR) (DBG OFF) (INLN).vi"("Input"=w515) -> ("Output"=w516:dbl)
                n297 = call "Math SubVI - Complex (PCR) (DBG OFF) (INLN).vi"("Input"=w516) -> ("Output"=w514:dbl)
              }
            }
            n298 = flat-sequence {
              tunnel: w499 -> [w513]
              tunnel: [w510] -> w498
              frame #0 {
                # "Repetition 3"
                n299 = call "Math SubVI - Simple (PCR) (DBG OFF) (INLN).vi"("Input"=w513) -> ("Output"=w511:dbl)
                n300 = call "Math SubVI - Medium (PCR) (DBG OFF) (INLN).vi"("Input"=w511) -> ("Output"=w512:dbl)
                n301 = call "Math SubVI - Complex (PCR) (DBG OFF) (INLN).vi"("Input"=w512) -> ("Output"=w510:dbl)
              }
            }
            n302 = flat-sequence {
              tunnel: w498 -> [w509]
              tunnel: [w506] -> w497
              frame #0 {
                # "Repetition 4"
                n303 = call "Math SubVI - Simple (PCR) (DBG OFF) (INLN).vi"("Input"=w509) -> ("Output"=w507:dbl)
                n304 = call "Math SubVI - Medium (PCR) (DBG OFF) (INLN).vi"("Input"=w507) -> ("Output"=w508:dbl)
                n305 = call "Math SubVI - Complex (PCR) (DBG OFF) (INLN).vi"("Input"=w508) -> ("Output"=w506:dbl)
              }
            }
            n306 = flat-sequence {
              tunnel: w497 -> [w505]
              tunnel: [w502] -> w496
              frame #0 {
                # "Repetition 5"
                n307 = call "Math SubVI - Simple (PCR) (DBG OFF) (INLN).vi"("Input"=w505) -> ("Output"=w503:dbl)
                n308 = call "Math SubVI - Medium (PCR) (DBG OFF) (INLN).vi"("Input"=w503) -> ("Output"=w504:dbl)
                n309 = call "Math SubVI - Complex (PCR) (DBG OFF) (INLN).vi"("Input"=w504) -> ("Output"=w502:dbl)
              }
            }
          }
        }
        n310 = local read "Stop VI?"() -> (w469:bool)
      }
      n311 = while "Loop 8" {
        tunnel: [w411] -> w46 mode=indexing
        tunnel: [w412] -> w47
        i -> [w412]
        stop <- w413 stop-if-true
        n312 = Random Number (0-1)() -> (number: 0 to 1=w410:dbl)
        n313 = disable-structure shown="Enabled" {
          disable-tunnel: w410 -> [w419 w445]
          disable-tunnel: [w418 w440] -> w411
          frame Disabled {
            # "Case 1: Subroutines"
            n314 = flat-sequence {
              tunnel: w419 -> [w439]
              tunnel: [w436] -> w414
              frame #0 {
                # "Repetition 1"
                n315 = call "Math SubVI - Simple (PCR) (DBG OFF) (SBRTN).vi"("Input"=w439) -> ("Output"=w437:dbl)
                n316 = call "Math SubVI - Medium (PCR) (DBG OFF) (SBRTN).vi"("Input"=w437) -> ("Output"=w438:dbl)
                n317 = call "Math SubVI - Complex (PCR) (DBG OFF) (SBRTN).vi"("Input"=w438) -> ("Output"=w436:dbl)
              }
            }
            n318 = flat-sequence {
              tunnel: w414 -> [w435]
              tunnel: [w432] -> w417
              frame #0 {
                # "Repetition 2"
                n319 = call "Math SubVI - Simple (PCR) (DBG OFF) (SBRTN).vi"("Input"=w435) -> ("Output"=w433:dbl)
                n320 = call "Math SubVI - Medium (PCR) (DBG OFF) (SBRTN).vi"("Input"=w433) -> ("Output"=w434:dbl)
                n321 = call "Math SubVI - Complex (PCR) (DBG OFF) (SBRTN).vi"("Input"=w434) -> ("Output"=w432:dbl)
              }
            }
            n322 = flat-sequence {
              tunnel: w417 -> [w431]
              tunnel: [w428] -> w416
              frame #0 {
                # "Repetition 3"
                n323 = call "Math SubVI - Simple (PCR) (DBG OFF) (SBRTN).vi"("Input"=w431) -> ("Output"=w429:dbl)
                n324 = call "Math SubVI - Medium (PCR) (DBG OFF) (SBRTN).vi"("Input"=w429) -> ("Output"=w430:dbl)
                n325 = call "Math SubVI - Complex (PCR) (DBG OFF) (SBRTN).vi"("Input"=w430) -> ("Output"=w428:dbl)
              }
            }
            n326 = flat-sequence {
              tunnel: w416 -> [w427]
              tunnel: [w424] -> w415
              frame #0 {
                # "Repetition 4"
                n327 = call "Math SubVI - Simple (PCR) (DBG OFF) (SBRTN).vi"("Input"=w427) -> ("Output"=w425:dbl)
                n328 = call "Math SubVI - Medium (PCR) (DBG OFF) (SBRTN).vi"("Input"=w425) -> ("Output"=w426:dbl)
                n329 = call "Math SubVI - Complex (PCR) (DBG OFF) (SBRTN).vi"("Input"=w426) -> ("Output"=w424:dbl)
              }
            }
            n330 = flat-sequence {
              tunnel: w415 -> [w423]
              tunnel: [w420] -> w418
              frame #0 {
                # "Repetition 5"
                n331 = call "Math SubVI - Simple (PCR) (DBG OFF) (SBRTN).vi"("Input"=w423) -> ("Output"=w421:dbl)
                n332 = call "Math SubVI - Medium (PCR) (DBG OFF) (SBRTN).vi"("Input"=w421) -> ("Output"=w422:dbl)
                n333 = call "Math SubVI - Complex (PCR) (DBG OFF) (SBRTN).vi"("Input"=w422) -> ("Output"=w420:dbl)
              }
            }
          }
          frame Enabled {
            # "Case 2: Inline VIs"
            n334 = flat-sequence {
              tunnel: w445 -> [w465]
              tunnel: [w462] -> w444
              frame #0 {
                # "Repetition 1"
                n335 = call "Math SubVI - Simple (PCR) (DBG OFF) (INLN).vi"("Input"=w465) -> ("Output"=w463:dbl)
                n336 = call "Math SubVI - Medium (PCR) (DBG OFF) (INLN).vi"("Input"=w463) -> ("Output"=w464:dbl)
                n337 = call "Math SubVI - Complex (PCR) (DBG OFF) (INLN).vi"("Input"=w464) -> ("Output"=w462:dbl)
              }
            }
            n338 = flat-sequence {
              tunnel: w444 -> [w461]
              tunnel: [w458] -> w443
              frame #0 {
                # "Repetition 2"
                n339 = call "Math SubVI - Simple (PCR) (DBG OFF) (INLN).vi"("Input"=w461) -> ("Output"=w459:dbl)
                n340 = call "Math SubVI - Medium (PCR) (DBG OFF) (INLN).vi"("Input"=w459) -> ("Output"=w460:dbl)
                n341 = call "Math SubVI - Complex (PCR) (DBG OFF) (INLN).vi"("Input"=w460) -> ("Output"=w458:dbl)
              }
            }
            n342 = flat-sequence {
              tunnel: w443 -> [w457]
              tunnel: [w454] -> w442
              frame #0 {
                # "Repetition 3"
                n343 = call "Math SubVI - Simple (PCR) (DBG OFF) (INLN).vi"("Input"=w457) -> ("Output"=w455:dbl)
                n344 = call "Math SubVI - Medium (PCR) (DBG OFF) (INLN).vi"("Input"=w455) -> ("Output"=w456:dbl)
                n345 = call "Math SubVI - Complex (PCR) (DBG OFF) (INLN).vi"("Input"=w456) -> ("Output"=w454:dbl)
              }
            }
            n346 = flat-sequence {
              tunnel: w442 -> [w453]
              tunnel: [w450] -> w441
              frame #0 {
                # "Repetition 4"
                n347 = call "Math SubVI - Simple (PCR) (DBG OFF) (INLN).vi"("Input"=w453) -> ("Output"=w451:dbl)
                n348 = call "Math SubVI - Medium (PCR) (DBG OFF) (INLN).vi"("Input"=w451) -> ("Output"=w452:dbl)
                n349 = call "Math SubVI - Complex (PCR) (DBG OFF) (INLN).vi"("Input"=w452) -> ("Output"=w450:dbl)
              }
            }
            n350 = flat-sequence {
              tunnel: w441 -> [w449]
              tunnel: [w446] -> w440
              frame #0 {
                # "Repetition 5"
                n351 = call "Math SubVI - Simple (PCR) (DBG OFF) (INLN).vi"("Input"=w449) -> ("Output"=w447:dbl)
                n352 = call "Math SubVI - Medium (PCR) (DBG OFF) (INLN).vi"("Input"=w447) -> ("Output"=w448:dbl)
                n353 = call "Math SubVI - Complex (PCR) (DBG OFF) (INLN).vi"("Input"=w448) -> ("Output"=w446:dbl)
              }
            }
          }
        }
        n354 = local read "Stop VI?"() -> (w413:bool)
      }
      n355 = while "Loop 9" {
        tunnel: [w355] -> w44 mode=indexing
        tunnel: [w356] -> w45
        i -> [w356]
        stop <- w357 stop-if-true
        n356 = Random Number (0-1)() -> (number: 0 to 1=w354:dbl)
        n357 = disable-structure shown="Enabled" {
          disable-tunnel: w354 -> [w363 w389]
          disable-tunnel: [w362 w384] -> w355
          frame Disabled {
            # "Case 1: Subroutines"
            n358 = flat-sequence {
              tunnel: w363 -> [w383]
              tunnel: [w380] -> w358
              frame #0 {
                # "Repetition 1"
                n359 = call "Math SubVI - Simple (PCR) (DBG OFF) (SBRTN).vi"("Input"=w383) -> ("Output"=w381:dbl)
                n360 = call "Math SubVI - Medium (PCR) (DBG OFF) (SBRTN).vi"("Input"=w381) -> ("Output"=w382:dbl)
                n361 = call "Math SubVI - Complex (PCR) (DBG OFF) (SBRTN).vi"("Input"=w382) -> ("Output"=w380:dbl)
              }
            }
            n362 = flat-sequence {
              tunnel: w358 -> [w379]
              tunnel: [w376] -> w361
              frame #0 {
                # "Repetition 2"
                n363 = call "Math SubVI - Simple (PCR) (DBG OFF) (SBRTN).vi"("Input"=w379) -> ("Output"=w377:dbl)
                n364 = call "Math SubVI - Medium (PCR) (DBG OFF) (SBRTN).vi"("Input"=w377) -> ("Output"=w378:dbl)
                n365 = call "Math SubVI - Complex (PCR) (DBG OFF) (SBRTN).vi"("Input"=w378) -> ("Output"=w376:dbl)
              }
            }
            n366 = flat-sequence {
              tunnel: w361 -> [w375]
              tunnel: [w372] -> w360
              frame #0 {
                # "Repetition 3"
                n367 = call "Math SubVI - Simple (PCR) (DBG OFF) (SBRTN).vi"("Input"=w375) -> ("Output"=w373:dbl)
                n368 = call "Math SubVI - Medium (PCR) (DBG OFF) (SBRTN).vi"("Input"=w373) -> ("Output"=w374:dbl)
                n369 = call "Math SubVI - Complex (PCR) (DBG OFF) (SBRTN).vi"("Input"=w374) -> ("Output"=w372:dbl)
              }
            }
            n370 = flat-sequence {
              tunnel: w360 -> [w371]
              tunnel: [w368] -> w359
              frame #0 {
                # "Repetition 4"
                n371 = call "Math SubVI - Simple (PCR) (DBG OFF) (SBRTN).vi"("Input"=w371) -> ("Output"=w369:dbl)
                n372 = call "Math SubVI - Medium (PCR) (DBG OFF) (SBRTN).vi"("Input"=w369) -> ("Output"=w370:dbl)
                n373 = call "Math SubVI - Complex (PCR) (DBG OFF) (SBRTN).vi"("Input"=w370) -> ("Output"=w368:dbl)
              }
            }
            n374 = flat-sequence {
              tunnel: w359 -> [w367]
              tunnel: [w364] -> w362
              frame #0 {
                # "Repetition 5"
                n375 = call "Math SubVI - Simple (PCR) (DBG OFF) (SBRTN).vi"("Input"=w367) -> ("Output"=w365:dbl)
                n376 = call "Math SubVI - Medium (PCR) (DBG OFF) (SBRTN).vi"("Input"=w365) -> ("Output"=w366:dbl)
                n377 = call "Math SubVI - Complex (PCR) (DBG OFF) (SBRTN).vi"("Input"=w366) -> ("Output"=w364:dbl)
              }
            }
          }
          frame Enabled {
            # "Case 2: Inline VIs"
            n378 = flat-sequence {
              tunnel: w389 -> [w409]
              tunnel: [w406] -> w388
              frame #0 {
                # "Repetition 1"
                n379 = call "Math SubVI - Simple (PCR) (DBG OFF) (INLN).vi"("Input"=w409) -> ("Output"=w407:dbl)
                n380 = call "Math SubVI - Medium (PCR) (DBG OFF) (INLN).vi"("Input"=w407) -> ("Output"=w408:dbl)
                n381 = call "Math SubVI - Complex (PCR) (DBG OFF) (INLN).vi"("Input"=w408) -> ("Output"=w406:dbl)
              }
            }
            n382 = flat-sequence {
              tunnel: w388 -> [w405]
              tunnel: [w402] -> w387
              frame #0 {
                # "Repetition 2"
                n383 = call "Math SubVI - Simple (PCR) (DBG OFF) (INLN).vi"("Input"=w405) -> ("Output"=w403:dbl)
                n384 = call "Math SubVI - Medium (PCR) (DBG OFF) (INLN).vi"("Input"=w403) -> ("Output"=w404:dbl)
                n385 = call "Math SubVI - Complex (PCR) (DBG OFF) (INLN).vi"("Input"=w404) -> ("Output"=w402:dbl)
              }
            }
            n386 = flat-sequence {
              tunnel: w387 -> [w401]
              tunnel: [w398] -> w386
              frame #0 {
                # "Repetition 3"
                n387 = call "Math SubVI - Simple (PCR) (DBG OFF) (INLN).vi"("Input"=w401) -> ("Output"=w399:dbl)
                n388 = call "Math SubVI - Medium (PCR) (DBG OFF) (INLN).vi"("Input"=w399) -> ("Output"=w400:dbl)
                n389 = call "Math SubVI - Complex (PCR) (DBG OFF) (INLN).vi"("Input"=w400) -> ("Output"=w398:dbl)
              }
            }
            n390 = flat-sequence {
              tunnel: w386 -> [w397]
              tunnel: [w394] -> w385
              frame #0 {
                # "Repetition 4"
                n391 = call "Math SubVI - Simple (PCR) (DBG OFF) (INLN).vi"("Input"=w397) -> ("Output"=w395:dbl)
                n392 = call "Math SubVI - Medium (PCR) (DBG OFF) (INLN).vi"("Input"=w395) -> ("Output"=w396:dbl)
                n393 = call "Math SubVI - Complex (PCR) (DBG OFF) (INLN).vi"("Input"=w396) -> ("Output"=w394:dbl)
              }
            }
            n394 = flat-sequence {
              tunnel: w385 -> [w393]
              tunnel: [w390] -> w384
              frame #0 {
                # "Repetition 5"
                n395 = call "Math SubVI - Simple (PCR) (DBG OFF) (INLN).vi"("Input"=w393) -> ("Output"=w391:dbl)
                n396 = call "Math SubVI - Medium (PCR) (DBG OFF) (INLN).vi"("Input"=w391) -> ("Output"=w392:dbl)
                n397 = call "Math SubVI - Complex (PCR) (DBG OFF) (INLN).vi"("Input"=w392) -> ("Output"=w390:dbl)
              }
            }
          }
        }
        n398 = local read "Stop VI?"() -> (w357:bool)
      }
      n399 = while "Loop 10" {
        tunnel: [w299] -> w42 mode=indexing
        tunnel: [w300] -> w43
        i -> [w300]
        stop <- w301 stop-if-true
        n400 = Random Number (0-1)() -> (number: 0 to 1=w298:dbl)
        n401 = disable-structure shown="Enabled" {
          disable-tunnel: w298 -> [w307 w333]
          disable-tunnel: [w306 w328] -> w299
          frame Disabled {
            # "Case 1: Subroutines"
            n402 = flat-sequence {
              tunnel: w307 -> [w327]
              tunnel: [w324] -> w302
              frame #0 {
                # "Repetition 1"
                n403 = call "Math SubVI - Simple (PCR) (DBG OFF) (SBRTN).vi"("Input"=w327) -> ("Output"=w325:dbl)
                n404 = call "Math SubVI - Medium (PCR) (DBG OFF) (SBRTN).vi"("Input"=w325) -> ("Output"=w326:dbl)
                n405 = call "Math SubVI - Complex (PCR) (DBG OFF) (SBRTN).vi"("Input"=w326) -> ("Output"=w324:dbl)
              }
            }
            n406 = flat-sequence {
              tunnel: w302 -> [w323]
              tunnel: [w320] -> w305
              frame #0 {
                # "Repetition 2"
                n407 = call "Math SubVI - Simple (PCR) (DBG OFF) (SBRTN).vi"("Input"=w323) -> ("Output"=w321:dbl)
                n408 = call "Math SubVI - Medium (PCR) (DBG OFF) (SBRTN).vi"("Input"=w321) -> ("Output"=w322:dbl)
                n409 = call "Math SubVI - Complex (PCR) (DBG OFF) (SBRTN).vi"("Input"=w322) -> ("Output"=w320:dbl)
              }
            }
            n410 = flat-sequence {
              tunnel: w305 -> [w319]
              tunnel: [w316] -> w304
              frame #0 {
                # "Repetition 3"
                n411 = call "Math SubVI - Simple (PCR) (DBG OFF) (SBRTN).vi"("Input"=w319) -> ("Output"=w317:dbl)
                n412 = call "Math SubVI - Medium (PCR) (DBG OFF) (SBRTN).vi"("Input"=w317) -> ("Output"=w318:dbl)
                n413 = call "Math SubVI - Complex (PCR) (DBG OFF) (SBRTN).vi"("Input"=w318) -> ("Output"=w316:dbl)
              }
            }
            n414 = flat-sequence {
              tunnel: w304 -> [w315]
              tunnel: [w312] -> w303
              frame #0 {
                # "Repetition 4"
                n415 = call "Math SubVI - Simple (PCR) (DBG OFF) (SBRTN).vi"("Input"=w315) -> ("Output"=w313:dbl)
                n416 = call "Math SubVI - Medium (PCR) (DBG OFF) (SBRTN).vi"("Input"=w313) -> ("Output"=w314:dbl)
                n417 = call "Math SubVI - Complex (PCR) (DBG OFF) (SBRTN).vi"("Input"=w314) -> ("Output"=w312:dbl)
              }
            }
            n418 = flat-sequence {
              tunnel: w303 -> [w311]
              tunnel: [w308] -> w306
              frame #0 {
                # "Repetition 5"
                n419 = call "Math SubVI - Simple (PCR) (DBG OFF) (SBRTN).vi"("Input"=w311) -> ("Output"=w309:dbl)
                n420 = call "Math SubVI - Medium (PCR) (DBG OFF) (SBRTN).vi"("Input"=w309) -> ("Output"=w310:dbl)
                n421 = call "Math SubVI - Complex (PCR) (DBG OFF) (SBRTN).vi"("Input"=w310) -> ("Output"=w308:dbl)
              }
            }
          }
          frame Enabled {
            # "Case 2: Inline VIs"
            n422 = flat-sequence {
              tunnel: w333 -> [w353]
              tunnel: [w350] -> w332
              frame #0 {
                # "Repetition 1"
                n423 = call "Math SubVI - Simple (PCR) (DBG OFF) (INLN).vi"("Input"=w353) -> ("Output"=w351:dbl)
                n424 = call "Math SubVI - Medium (PCR) (DBG OFF) (INLN).vi"("Input"=w351) -> ("Output"=w352:dbl)
                n425 = call "Math SubVI - Complex (PCR) (DBG OFF) (INLN).vi"("Input"=w352) -> ("Output"=w350:dbl)
              }
            }
            n426 = flat-sequence {
              tunnel: w332 -> [w349]
              tunnel: [w346] -> w331
              frame #0 {
                # "Repetition 2"
                n427 = call "Math SubVI - Simple (PCR) (DBG OFF) (INLN).vi"("Input"=w349) -> ("Output"=w347:dbl)
                n428 = call "Math SubVI - Medium (PCR) (DBG OFF) (INLN).vi"("Input"=w347) -> ("Output"=w348:dbl)
                n429 = call "Math SubVI - Complex (PCR) (DBG OFF) (INLN).vi"("Input"=w348) -> ("Output"=w346:dbl)
              }
            }
            n430 = flat-sequence {
              tunnel: w331 -> [w345]
              tunnel: [w342] -> w330
              frame #0 {
                # "Repetition 3"
                n431 = call "Math SubVI - Simple (PCR) (DBG OFF) (INLN).vi"("Input"=w345) -> ("Output"=w343:dbl)
                n432 = call "Math SubVI - Medium (PCR) (DBG OFF) (INLN).vi"("Input"=w343) -> ("Output"=w344:dbl)
                n433 = call "Math SubVI - Complex (PCR) (DBG OFF) (INLN).vi"("Input"=w344) -> ("Output"=w342:dbl)
              }
            }
            n434 = flat-sequence {
              tunnel: w330 -> [w341]
              tunnel: [w338] -> w329
              frame #0 {
                # "Repetition 4"
                n435 = call "Math SubVI - Simple (PCR) (DBG OFF) (INLN).vi"("Input"=w341) -> ("Output"=w339:dbl)
                n436 = call "Math SubVI - Medium (PCR) (DBG OFF) (INLN).vi"("Input"=w339) -> ("Output"=w340:dbl)
                n437 = call "Math SubVI - Complex (PCR) (DBG OFF) (INLN).vi"("Input"=w340) -> ("Output"=w338:dbl)
              }
            }
            n438 = flat-sequence {
              tunnel: w329 -> [w337]
              tunnel: [w334] -> w328
              frame #0 {
                # "Repetition 5"
                n439 = call "Math SubVI - Simple (PCR) (DBG OFF) (INLN).vi"("Input"=w337) -> ("Output"=w335:dbl)
                n440 = call "Math SubVI - Medium (PCR) (DBG OFF) (INLN).vi"("Input"=w335) -> ("Output"=w336:dbl)
                n441 = call "Math SubVI - Complex (PCR) (DBG OFF) (INLN).vi"("Input"=w336) -> ("Output"=w334:dbl)
              }
            }
          }
        }
        n442 = local read "Stop VI?"() -> (w301:bool)
      }
      n443 = while "Loop 11" {
        tunnel: [w243] -> w41 mode=indexing
        tunnel: [w244] -> w40
        i -> [w244]
        stop <- w245 stop-if-true
        n444 = Random Number (0-1)() -> (number: 0 to 1=w242:dbl)
        n445 = disable-structure shown="Enabled" {
          disable-tunnel: w242 -> [w251 w277]
          disable-tunnel: [w250 w272] -> w243
          frame Disabled {
            # "Case 1: Subroutines"
            n446 = flat-sequence {
              tunnel: w251 -> [w271]
              tunnel: [w268] -> w246
              frame #0 {
                # "Repetition 1"
                n447 = call "Math SubVI - Simple (PCR) (DBG OFF) (SBRTN).vi"("Input"=w271) -> ("Output"=w269:dbl)
                n448 = call "Math SubVI - Medium (PCR) (DBG OFF) (SBRTN).vi"("Input"=w269) -> ("Output"=w270:dbl)
                n449 = call "Math SubVI - Complex (PCR) (DBG OFF) (SBRTN).vi"("Input"=w270) -> ("Output"=w268:dbl)
              }
            }
            n450 = flat-sequence {
              tunnel: w246 -> [w267]
              tunnel: [w264] -> w249
              frame #0 {
                # "Repetition 2"
                n451 = call "Math SubVI - Simple (PCR) (DBG OFF) (SBRTN).vi"("Input"=w267) -> ("Output"=w265:dbl)
                n452 = call "Math SubVI - Medium (PCR) (DBG OFF) (SBRTN).vi"("Input"=w265) -> ("Output"=w266:dbl)
                n453 = call "Math SubVI - Complex (PCR) (DBG OFF) (SBRTN).vi"("Input"=w266) -> ("Output"=w264:dbl)
              }
            }
            n454 = flat-sequence {
              tunnel: w249 -> [w263]
              tunnel: [w260] -> w248
              frame #0 {
                # "Repetition 3"
                n455 = call "Math SubVI - Simple (PCR) (DBG OFF) (SBRTN).vi"("Input"=w263) -> ("Output"=w261:dbl)
                n456 = call "Math SubVI - Medium (PCR) (DBG OFF) (SBRTN).vi"("Input"=w261) -> ("Output"=w262:dbl)
                n457 = call "Math SubVI - Complex (PCR) (DBG OFF) (SBRTN).vi"("Input"=w262) -> ("Output"=w260:dbl)
              }
            }
            n458 = flat-sequence {
              tunnel: w248 -> [w259]
              tunnel: [w256] -> w247
              frame #0 {
                # "Repetition 4"
                n459 = call "Math SubVI - Simple (PCR) (DBG OFF) (SBRTN).vi"("Input"=w259) -> ("Output"=w257:dbl)
                n460 = call "Math SubVI - Medium (PCR) (DBG OFF) (SBRTN).vi"("Input"=w257) -> ("Output"=w258:dbl)
                n461 = call "Math SubVI - Complex (PCR) (DBG OFF) (SBRTN).vi"("Input"=w258) -> ("Output"=w256:dbl)
              }
            }
            n462 = flat-sequence {
              tunnel: w247 -> [w255]
              tunnel: [w252] -> w250
              frame #0 {
                # "Repetition 5"
                n463 = call "Math SubVI - Simple (PCR) (DBG OFF) (SBRTN).vi"("Input"=w255) -> ("Output"=w253:dbl)
                n464 = call "Math SubVI - Medium (PCR) (DBG OFF) (SBRTN).vi"("Input"=w253) -> ("Output"=w254:dbl)
                n465 = call "Math SubVI - Complex (PCR) (DBG OFF) (SBRTN).vi"("Input"=w254) -> ("Output"=w252:dbl)
              }
            }
          }
          frame Enabled {
            # "Case 2: Inline VIs"
            n466 = flat-sequence {
              tunnel: w277 -> [w297]
              tunnel: [w294] -> w276
              frame #0 {
                # "Repetition 1"
                n467 = call "Math SubVI - Simple (PCR) (DBG OFF) (INLN).vi"("Input"=w297) -> ("Output"=w295:dbl)
                n468 = call "Math SubVI - Medium (PCR) (DBG OFF) (INLN).vi"("Input"=w295) -> ("Output"=w296:dbl)
                n469 = call "Math SubVI - Complex (PCR) (DBG OFF) (INLN).vi"("Input"=w296) -> ("Output"=w294:dbl)
              }
            }
            n470 = flat-sequence {
              tunnel: w276 -> [w293]
              tunnel: [w290] -> w275
              frame #0 {
                # "Repetition 2"
                n471 = call "Math SubVI - Simple (PCR) (DBG OFF) (INLN).vi"("Input"=w293) -> ("Output"=w291:dbl)
                n472 = call "Math SubVI - Medium (PCR) (DBG OFF) (INLN).vi"("Input"=w291) -> ("Output"=w292:dbl)
                n473 = call "Math SubVI - Complex (PCR) (DBG OFF) (INLN).vi"("Input"=w292) -> ("Output"=w290:dbl)
              }
            }
            n474 = flat-sequence {
              tunnel: w275 -> [w289]
              tunnel: [w286] -> w274
              frame #0 {
                # "Repetition 3"
                n475 = call "Math SubVI - Simple (PCR) (DBG OFF) (INLN).vi"("Input"=w289) -> ("Output"=w287:dbl)
                n476 = call "Math SubVI - Medium (PCR) (DBG OFF) (INLN).vi"("Input"=w287) -> ("Output"=w288:dbl)
                n477 = call "Math SubVI - Complex (PCR) (DBG OFF) (INLN).vi"("Input"=w288) -> ("Output"=w286:dbl)
              }
            }
            n478 = flat-sequence {
              tunnel: w274 -> [w285]
              tunnel: [w282] -> w273
              frame #0 {
                # "Repetition 4"
                n479 = call "Math SubVI - Simple (PCR) (DBG OFF) (INLN).vi"("Input"=w285) -> ("Output"=w283:dbl)
                n480 = call "Math SubVI - Medium (PCR) (DBG OFF) (INLN).vi"("Input"=w283) -> ("Output"=w284:dbl)
                n481 = call "Math SubVI - Complex (PCR) (DBG OFF) (INLN).vi"("Input"=w284) -> ("Output"=w282:dbl)
              }
            }
            n482 = flat-sequence {
              tunnel: w273 -> [w281]
              tunnel: [w278] -> w272
              frame #0 {
                # "Repetition 5"
                n483 = call "Math SubVI - Simple (PCR) (DBG OFF) (INLN).vi"("Input"=w281) -> ("Output"=w279:dbl)
                n484 = call "Math SubVI - Medium (PCR) (DBG OFF) (INLN).vi"("Input"=w279) -> ("Output"=w280:dbl)
                n485 = call "Math SubVI - Complex (PCR) (DBG OFF) (INLN).vi"("Input"=w280) -> ("Output"=w278:dbl)
              }
            }
          }
        }
        n486 = local read "Stop VI?"() -> (w245:bool)
      }
      n487 = while "Loop 12" {
        tunnel: [w187] -> w38 mode=indexing
        tunnel: [w188] -> w37
        i -> [w188]
        stop <- w189 stop-if-true
        n488 = Random Number (0-1)() -> (number: 0 to 1=w186:dbl)
        n489 = disable-structure shown="Enabled" {
          disable-tunnel: w186 -> [w195 w221]
          disable-tunnel: [w194 w216] -> w187
          frame Disabled {
            # "Case 1: Subroutines"
            n490 = flat-sequence {
              tunnel: w195 -> [w215]
              tunnel: [w212] -> w190
              frame #0 {
                # "Repetition 1"
                n491 = call "Math SubVI - Simple (PCR) (DBG OFF) (SBRTN).vi"("Input"=w215) -> ("Output"=w213:dbl)
                n492 = call "Math SubVI - Medium (PCR) (DBG OFF) (SBRTN).vi"("Input"=w213) -> ("Output"=w214:dbl)
                n493 = call "Math SubVI - Complex (PCR) (DBG OFF) (SBRTN).vi"("Input"=w214) -> ("Output"=w212:dbl)
              }
            }
            n494 = flat-sequence {
              tunnel: w190 -> [w211]
              tunnel: [w208] -> w193
              frame #0 {
                # "Repetition 2"
                n495 = call "Math SubVI - Simple (PCR) (DBG OFF) (SBRTN).vi"("Input"=w211) -> ("Output"=w209:dbl)
                n496 = call "Math SubVI - Medium (PCR) (DBG OFF) (SBRTN).vi"("Input"=w209) -> ("Output"=w210:dbl)
                n497 = call "Math SubVI - Complex (PCR) (DBG OFF) (SBRTN).vi"("Input"=w210) -> ("Output"=w208:dbl)
              }
            }
            n498 = flat-sequence {
              tunnel: w193 -> [w207]
              tunnel: [w204] -> w192
              frame #0 {
                # "Repetition 3"
                n499 = call "Math SubVI - Simple (PCR) (DBG OFF) (SBRTN).vi"("Input"=w207) -> ("Output"=w205:dbl)
                n500 = call "Math SubVI - Medium (PCR) (DBG OFF) (SBRTN).vi"("Input"=w205) -> ("Output"=w206:dbl)
                n501 = call "Math SubVI - Complex (PCR) (DBG OFF) (SBRTN).vi"("Input"=w206) -> ("Output"=w204:dbl)
              }
            }
            n502 = flat-sequence {
              tunnel: w192 -> [w203]
              tunnel: [w200] -> w191
              frame #0 {
                # "Repetition 4"
                n503 = call "Math SubVI - Simple (PCR) (DBG OFF) (SBRTN).vi"("Input"=w203) -> ("Output"=w201:dbl)
                n504 = call "Math SubVI - Medium (PCR) (DBG OFF) (SBRTN).vi"("Input"=w201) -> ("Output"=w202:dbl)
                n505 = call "Math SubVI - Complex (PCR) (DBG OFF) (SBRTN).vi"("Input"=w202) -> ("Output"=w200:dbl)
              }
            }
            n506 = flat-sequence {
              tunnel: w191 -> [w199]
              tunnel: [w196] -> w194
              frame #0 {
                # "Repetition 5"
                n507 = call "Math SubVI - Simple (PCR) (DBG OFF) (SBRTN).vi"("Input"=w199) -> ("Output"=w197:dbl)
                n508 = call "Math SubVI - Medium (PCR) (DBG OFF) (SBRTN).vi"("Input"=w197) -> ("Output"=w198:dbl)
                n509 = call "Math SubVI - Complex (PCR) (DBG OFF) (SBRTN).vi"("Input"=w198) -> ("Output"=w196:dbl)
              }
            }
          }
          frame Enabled {
            # "Case 2: Inline VIs"
            n510 = flat-sequence {
              tunnel: w221 -> [w241]
              tunnel: [w238] -> w220
              frame #0 {
                # "Repetition 1"
                n511 = call "Math SubVI - Simple (PCR) (DBG OFF) (INLN).vi"("Input"=w241) -> ("Output"=w239:dbl)
                n512 = call "Math SubVI - Medium (PCR) (DBG OFF) (INLN).vi"("Input"=w239) -> ("Output"=w240:dbl)
                n513 = call "Math SubVI - Complex (PCR) (DBG OFF) (INLN).vi"("Input"=w240) -> ("Output"=w238:dbl)
              }
            }
            n514 = flat-sequence {
              tunnel: w220 -> [w237]
              tunnel: [w234] -> w219
              frame #0 {
                # "Repetition 2"
                n515 = call "Math SubVI - Simple (PCR) (DBG OFF) (INLN).vi"("Input"=w237) -> ("Output"=w235:dbl)
                n516 = call "Math SubVI - Medium (PCR) (DBG OFF) (INLN).vi"("Input"=w235) -> ("Output"=w236:dbl)
                n517 = call "Math SubVI - Complex (PCR) (DBG OFF) (INLN).vi"("Input"=w236) -> ("Output"=w234:dbl)
              }
            }
            n518 = flat-sequence {
              tunnel: w219 -> [w233]
              tunnel: [w230] -> w218
              frame #0 {
                # "Repetition 3"
                n519 = call "Math SubVI - Simple (PCR) (DBG OFF) (INLN).vi"("Input"=w233) -> ("Output"=w231:dbl)
                n520 = call "Math SubVI - Medium (PCR) (DBG OFF) (INLN).vi"("Input"=w231) -> ("Output"=w232:dbl)
                n521 = call "Math SubVI - Complex (PCR) (DBG OFF) (INLN).vi"("Input"=w232) -> ("Output"=w230:dbl)
              }
            }
            n522 = flat-sequence {
              tunnel: w218 -> [w229]
              tunnel: [w226] -> w217
              frame #0 {
                # "Repetition 4"
                n523 = call "Math SubVI - Simple (PCR) (DBG OFF) (INLN).vi"("Input"=w229) -> ("Output"=w227:dbl)
                n524 = call "Math SubVI - Medium (PCR) (DBG OFF) (INLN).vi"("Input"=w227) -> ("Output"=w228:dbl)
                n525 = call "Math SubVI - Complex (PCR) (DBG OFF) (INLN).vi"("Input"=w228) -> ("Output"=w226:dbl)
              }
            }
            n526 = flat-sequence {
              tunnel: w217 -> [w225]
              tunnel: [w222] -> w216
              frame #0 {
                # "Repetition 5"
                n527 = call "Math SubVI - Simple (PCR) (DBG OFF) (INLN).vi"("Input"=w225) -> ("Output"=w223:dbl)
                n528 = call "Math SubVI - Medium (PCR) (DBG OFF) (INLN).vi"("Input"=w223) -> ("Output"=w224:dbl)
                n529 = call "Math SubVI - Complex (PCR) (DBG OFF) (INLN).vi"("Input"=w224) -> ("Output"=w222:dbl)
              }
            }
          }
        }
        n530 = local read "Stop VI?"() -> (w189:bool)
      }
      n531 = while "Loop 13" {
        tunnel: [w131] -> w36 mode=indexing
        tunnel: [w132] -> w35
        i -> [w132]
        stop <- w133 stop-if-true
        n532 = Random Number (0-1)() -> (number: 0 to 1=w130:dbl)
        n533 = disable-structure shown="Enabled" {
          disable-tunnel: w130 -> [w139 w165]
          disable-tunnel: [w138 w160] -> w131
          frame Disabled {
            # "Case 1: Subroutines"
            n534 = flat-sequence {
              tunnel: w139 -> [w159]
              tunnel: [w156] -> w134
              frame #0 {
                # "Repetition 1"
                n535 = call "Math SubVI - Simple (PCR) (DBG OFF) (SBRTN).vi"("Input"=w159) -> ("Output"=w157:dbl)
                n536 = call "Math SubVI - Medium (PCR) (DBG OFF) (SBRTN).vi"("Input"=w157) -> ("Output"=w158:dbl)
                n537 = call "Math SubVI - Complex (PCR) (DBG OFF) (SBRTN).vi"("Input"=w158) -> ("Output"=w156:dbl)
              }
            }
            n538 = flat-sequence {
              tunnel: w134 -> [w155]
              tunnel: [w152] -> w137
              frame #0 {
                # "Repetition 2"
                n539 = call "Math SubVI - Simple (PCR) (DBG OFF) (SBRTN).vi"("Input"=w155) -> ("Output"=w153:dbl)
                n540 = call "Math SubVI - Medium (PCR) (DBG OFF) (SBRTN).vi"("Input"=w153) -> ("Output"=w154:dbl)
                n541 = call "Math SubVI - Complex (PCR) (DBG OFF) (SBRTN).vi"("Input"=w154) -> ("Output"=w152:dbl)
              }
            }
            n542 = flat-sequence {
              tunnel: w137 -> [w151]
              tunnel: [w148] -> w136
              frame #0 {
                # "Repetition 3"
                n543 = call "Math SubVI - Simple (PCR) (DBG OFF) (SBRTN).vi"("Input"=w151) -> ("Output"=w149:dbl)
                n544 = call "Math SubVI - Medium (PCR) (DBG OFF) (SBRTN).vi"("Input"=w149) -> ("Output"=w150:dbl)
                n545 = call "Math SubVI - Complex (PCR) (DBG OFF) (SBRTN).vi"("Input"=w150) -> ("Output"=w148:dbl)
              }
            }
            n546 = flat-sequence {
              tunnel: w136 -> [w147]
              tunnel: [w144] -> w135
              frame #0 {
                # "Repetition 4"
                n547 = call "Math SubVI - Simple (PCR) (DBG OFF) (SBRTN).vi"("Input"=w147) -> ("Output"=w145:dbl)
                n548 = call "Math SubVI - Medium (PCR) (DBG OFF) (SBRTN).vi"("Input"=w145) -> ("Output"=w146:dbl)
                n549 = call "Math SubVI - Complex (PCR) (DBG OFF) (SBRTN).vi"("Input"=w146) -> ("Output"=w144:dbl)
              }
            }
            n550 = flat-sequence {
              tunnel: w135 -> [w143]
              tunnel: [w140] -> w138
              frame #0 {
                # "Repetition 5"
                n551 = call "Math SubVI - Simple (PCR) (DBG OFF) (SBRTN).vi"("Input"=w143) -> ("Output"=w141:dbl)
                n552 = call "Math SubVI - Medium (PCR) (DBG OFF) (SBRTN).vi"("Input"=w141) -> ("Output"=w142:dbl)
                n553 = call "Math SubVI - Complex (PCR) (DBG OFF) (SBRTN).vi"("Input"=w142) -> ("Output"=w140:dbl)
              }
            }
          }
          frame Enabled {
            # "Case 2: Inline VIs"
            n554 = flat-sequence {
              tunnel: w165 -> [w185]
              tunnel: [w182] -> w164
              frame #0 {
                # "Repetition 1"
                n555 = call "Math SubVI - Simple (PCR) (DBG OFF) (INLN).vi"("Input"=w185) -> ("Output"=w183:dbl)
                n556 = call "Math SubVI - Medium (PCR) (DBG OFF) (INLN).vi"("Input"=w183) -> ("Output"=w184:dbl)
                n557 = call "Math SubVI - Complex (PCR) (DBG OFF) (INLN).vi"("Input"=w184) -> ("Output"=w182:dbl)
              }
            }
            n558 = flat-sequence {
              tunnel: w164 -> [w181]
              tunnel: [w178] -> w163
              frame #0 {
                # "Repetition 2"
                n559 = call "Math SubVI - Simple (PCR) (DBG OFF) (INLN).vi"("Input"=w181) -> ("Output"=w179:dbl)
                n560 = call "Math SubVI - Medium (PCR) (DBG OFF) (INLN).vi"("Input"=w179) -> ("Output"=w180:dbl)
                n561 = call "Math SubVI - Complex (PCR) (DBG OFF) (INLN).vi"("Input"=w180) -> ("Output"=w178:dbl)
              }
            }
            n562 = flat-sequence {
              tunnel: w163 -> [w177]
              tunnel: [w174] -> w162
              frame #0 {
                # "Repetition 3"
                n563 = call "Math SubVI - Simple (PCR) (DBG OFF) (INLN).vi"("Input"=w177) -> ("Output"=w175:dbl)
                n564 = call "Math SubVI - Medium (PCR) (DBG OFF) (INLN).vi"("Input"=w175) -> ("Output"=w176:dbl)
                n565 = call "Math SubVI - Complex (PCR) (DBG OFF) (INLN).vi"("Input"=w176) -> ("Output"=w174:dbl)
              }
            }
            n566 = flat-sequence {
              tunnel: w162 -> [w173]
              tunnel: [w170] -> w161
              frame #0 {
                # "Repetition 4"
                n567 = call "Math SubVI - Simple (PCR) (DBG OFF) (INLN).vi"("Input"=w173) -> ("Output"=w171:dbl)
                n568 = call "Math SubVI - Medium (PCR) (DBG OFF) (INLN).vi"("Input"=w171) -> ("Output"=w172:dbl)
                n569 = call "Math SubVI - Complex (PCR) (DBG OFF) (INLN).vi"("Input"=w172) -> ("Output"=w170:dbl)
              }
            }
            n570 = flat-sequence {
              tunnel: w161 -> [w169]
              tunnel: [w166] -> w160
              frame #0 {
                # "Repetition 5"
                n571 = call "Math SubVI - Simple (PCR) (DBG OFF) (INLN).vi"("Input"=w169) -> ("Output"=w167:dbl)
                n572 = call "Math SubVI - Medium (PCR) (DBG OFF) (INLN).vi"("Input"=w167) -> ("Output"=w168:dbl)
                n573 = call "Math SubVI - Complex (PCR) (DBG OFF) (INLN).vi"("Input"=w168) -> ("Output"=w166:dbl)
              }
            }
          }
        }
        n574 = local read "Stop VI?"() -> (w133:bool)
      }
      n575 = while "Loop 14" {
        tunnel: [w75] -> w34 mode=indexing
        tunnel: [w76] -> w33
        i -> [w76]
        stop <- w77 stop-if-true
        n576 = Random Number (0-1)() -> (number: 0 to 1=w74:dbl)
        n577 = disable-structure shown="Enabled" {
          disable-tunnel: w74 -> [w83 w109]
          disable-tunnel: [w82 w104] -> w75
          frame Disabled {
            # "Case 1: Subroutines"
            n578 = flat-sequence {
              tunnel: w83 -> [w103]
              tunnel: [w100] -> w78
              frame #0 {
                # "Repetition 1"
                n579 = call "Math SubVI - Simple (PCR) (DBG OFF) (SBRTN).vi"("Input"=w103) -> ("Output"=w101:dbl)
                n580 = call "Math SubVI - Medium (PCR) (DBG OFF) (SBRTN).vi"("Input"=w101) -> ("Output"=w102:dbl)
                n581 = call "Math SubVI - Complex (PCR) (DBG OFF) (SBRTN).vi"("Input"=w102) -> ("Output"=w100:dbl)
              }
            }
            n582 = flat-sequence {
              tunnel: w78 -> [w99]
              tunnel: [w96] -> w81
              frame #0 {
                # "Repetition 2"
                n583 = call "Math SubVI - Simple (PCR) (DBG OFF) (SBRTN).vi"("Input"=w99) -> ("Output"=w97:dbl)
                n584 = call "Math SubVI - Medium (PCR) (DBG OFF) (SBRTN).vi"("Input"=w97) -> ("Output"=w98:dbl)
                n585 = call "Math SubVI - Complex (PCR) (DBG OFF) (SBRTN).vi"("Input"=w98) -> ("Output"=w96:dbl)
              }
            }
            n586 = flat-sequence {
              tunnel: w81 -> [w95]
              tunnel: [w92] -> w80
              frame #0 {
                # "Repetition 3"
                n587 = call "Math SubVI - Simple (PCR) (DBG OFF) (SBRTN).vi"("Input"=w95) -> ("Output"=w93:dbl)
                n588 = call "Math SubVI - Medium (PCR) (DBG OFF) (SBRTN).vi"("Input"=w93) -> ("Output"=w94:dbl)
                n589 = call "Math SubVI - Complex (PCR) (DBG OFF) (SBRTN).vi"("Input"=w94) -> ("Output"=w92:dbl)
              }
            }
            n590 = flat-sequence {
              tunnel: w80 -> [w91]
              tunnel: [w88] -> w79
              frame #0 {
                # "Repetition 4"
                n591 = call "Math SubVI - Simple (PCR) (DBG OFF) (SBRTN).vi"("Input"=w91) -> ("Output"=w89:dbl)
                n592 = call "Math SubVI - Medium (PCR) (DBG OFF) (SBRTN).vi"("Input"=w89) -> ("Output"=w90:dbl)
                n593 = call "Math SubVI - Complex (PCR) (DBG OFF) (SBRTN).vi"("Input"=w90) -> ("Output"=w88:dbl)
              }
            }
            n594 = flat-sequence {
              tunnel: w79 -> [w87]
              tunnel: [w84] -> w82
              frame #0 {
                # "Repetition 5"
                n595 = call "Math SubVI - Simple (PCR) (DBG OFF) (SBRTN).vi"("Input"=w87) -> ("Output"=w85:dbl)
                n596 = call "Math SubVI - Medium (PCR) (DBG OFF) (SBRTN).vi"("Input"=w85) -> ("Output"=w86:dbl)
                n597 = call "Math SubVI - Complex (PCR) (DBG OFF) (SBRTN).vi"("Input"=w86) -> ("Output"=w84:dbl)
              }
            }
          }
          frame Enabled {
            # "Case 2: Inline VIs"
            n598 = flat-sequence {
              tunnel: w109 -> [w129]
              tunnel: [w126] -> w108
              frame #0 {
                # "Repetition 1"
                n599 = call "Math SubVI - Simple (PCR) (DBG OFF) (INLN).vi"("Input"=w129) -> ("Output"=w127:dbl)
                n600 = call "Math SubVI - Medium (PCR) (DBG OFF) (INLN).vi"("Input"=w127) -> ("Output"=w128:dbl)
                n601 = call "Math SubVI - Complex (PCR) (DBG OFF) (INLN).vi"("Input"=w128) -> ("Output"=w126:dbl)
              }
            }
            n602 = flat-sequence {
              tunnel: w108 -> [w125]
              tunnel: [w122] -> w107
              frame #0 {
                # "Repetition 2"
                n603 = call "Math SubVI - Simple (PCR) (DBG OFF) (INLN).vi"("Input"=w125) -> ("Output"=w123:dbl)
                n604 = call "Math SubVI - Medium (PCR) (DBG OFF) (INLN).vi"("Input"=w123) -> ("Output"=w124:dbl)
                n605 = call "Math SubVI - Complex (PCR) (DBG OFF) (INLN).vi"("Input"=w124) -> ("Output"=w122:dbl)
              }
            }
            n606 = flat-sequence {
              tunnel: w107 -> [w121]
              tunnel: [w118] -> w106
              frame #0 {
                # "Repetition 3"
                n607 = call "Math SubVI - Simple (PCR) (DBG OFF) (INLN).vi"("Input"=w121) -> ("Output"=w119:dbl)
                n608 = call "Math SubVI - Medium (PCR) (DBG OFF) (INLN).vi"("Input"=w119) -> ("Output"=w120:dbl)
                n609 = call "Math SubVI - Complex (PCR) (DBG OFF) (INLN).vi"("Input"=w120) -> ("Output"=w118:dbl)
              }
            }
            n610 = flat-sequence {
              tunnel: w106 -> [w117]
              tunnel: [w114] -> w105
              frame #0 {
                # "Repetition 4"
                n611 = call "Math SubVI - Simple (PCR) (DBG OFF) (INLN).vi"("Input"=w117) -> ("Output"=w115:dbl)
                n612 = call "Math SubVI - Medium (PCR) (DBG OFF) (INLN).vi"("Input"=w115) -> ("Output"=w116:dbl)
                n613 = call "Math SubVI - Complex (PCR) (DBG OFF) (INLN).vi"("Input"=w116) -> ("Output"=w114:dbl)
              }
            }
            n614 = flat-sequence {
              tunnel: w105 -> [w113]
              tunnel: [w110] -> w104
              frame #0 {
                # "Repetition 5"
                n615 = call "Math SubVI - Simple (PCR) (DBG OFF) (INLN).vi"("Input"=w113) -> ("Output"=w111:dbl)
                n616 = call "Math SubVI - Medium (PCR) (DBG OFF) (INLN).vi"("Input"=w111) -> ("Output"=w112:dbl)
                n617 = call "Math SubVI - Complex (PCR) (DBG OFF) (INLN).vi"("Input"=w112) -> ("Output"=w110:dbl)
              }
            }
          }
        }
        n618 = local read "Stop VI?"() -> (w77:bool)
      }
      n619 = call <vilib>:"High Resolution Polling Wait.vi"("seconds to wait"=w73) -> ("error out"=w72:errorcluster)  [unwired: 10 in]
      n620 = flat-sequence {
        tunnel: w72 -> [w858]
        frame #0 {
          n621 = call <vilib>:"Clear Errors.vi"("error in (no error)"=w858) -> ()  [unwired: 5 in, 2 out]
          "Stop VI?" <- TRUE
        }
      }
      n622 = Increment(x=w52) -> (x+1=w65:i32)
      n623 = Increment(x=w50) -> (x+1=w60:i32)
      n624 = Increment(x=w48) -> (x+1=w61:i32)
      n625 = Increment(x=w47) -> (x+1=w62:i32)
      n626 = Increment(x=w45) -> (x+1=w63:i32)
      n627 = Increment(x=w43) -> (x+1=w64:i32)
      n628 = Increment(x=w40) -> (x+1=w39:i32)
      n629 = Increment(x=w37) -> (x+1=w32:i32)
      n630 = Increment(x=w35) -> (x+1=w31:i32)
      n631 = Increment(x=w33) -> (x+1=w30:i32)
      n632 = Increment(x=w70) -> (x+1=w69:i32)
      n633 = Increment(x=w58) -> (x+1=w68:i32)
      n634 = Increment(x=w56) -> (x+1=w67:i32)
      n635 = Increment(x=w54) -> (x+1=w66:i32)
    }
    frame #2 {
      n636 = Build Array(w892, w891, w887, w886, w878, w877, w876, w875, w874, w873, w863, w862, w861, w860) -> (w872:i32[])
      n637 = for {
        tunnel: w872 -> [w898] mode=indexing
        tunnel: [w897] -> w871 mode=indexing
        n638 = Number To Decimal String(number=w898) -> (decimal integer string=w897:string)  [unwired: 1 in]
      }
      n639 = To Double Precision Float(number=w872) -> (double precision float=w885:dbl[])
      n640 = call-poly <vilib>:"Mean.vi"("X"=w885) -> ("mean"=w890:dbl)  [unwired: 1 out]
      "Avg. No. Of Iterations Executed - All Loops" <- w890
      n641 = disable-structure shown="Enabled" {
        disable-tunnel: w890 -> [w896 _]
        frame Disabled {
          n642 = call "Copy Result To Clipboard.vi"("No. Of Decimal Places (6)"=u32 1, "Input"=w896) -> ()
        }
        frame Enabled {
        }
      }
      n643 = call-poly <vilib>:"1D String Array to Delimited String.vi"("delimiter"="\r\n", "string array"=w871) -> ("delimited string"=w868:string)  [unwired: 9 in]
      "No. Of Iterations As Block Of Text (easy to copy into Excel)" <- w868
      n644 = invoke class="Application" method="Clipboard.Write"("Param 0"=w868) -> (error out=w869:errorcluster)  [unwired: 3 in, 3 out]
      n645 = call <vilib>:"Clear Errors.vi"("error in (no error)"=w869) -> ()  [unwired: 5 in, 2 out]
      "No. Of Iterations Executed - Loop 1" <- w892
      "Output - Loop 1" <- w894
      "No. Of Iterations Executed - Loop 2" <- w891
      "Output - Loop 2" <- w893
      "No. Of Iterations Executed - Loop 3" <- w887
      "Output - Loop 3" <- w889
      "No. Of Iterations Executed - Loop 4" <- w886
      "Output - Loop 4" <- w888
      "No. Of Iterations Executed - Loop 5" <- w878
      "Output - Loop 5" <- w884
      "No. Of Iterations Executed - Loop 6" <- w877
      "Output - Loop 6" <- w883
      "No. Of Iterations Executed - Loop 7" <- w876
      "Output - Loop 7" <- w882
      "No. Of Iterations Executed - Loop 8" <- w875
      "Output - Loop 8" <- w881
      "No. Of Iterations Executed - Loop 9" <- w874
      "Output - Loop 9" <- w880
      "No. Of Iterations Executed - Loop 10" <- w873
      "Output - Loop 10" <- w879
      "No. Of Iterations Executed - Loop 11" <- w863
      "Output - Loop 11" <- w867
      "No. Of Iterations Executed - Loop 12" <- w862
      "Output - Loop 12" <- w866
      "No. Of Iterations Executed - Loop 13" <- w861
      "Output - Loop 13" <- w865
      "No. Of Iterations Executed - Loop 14" <- w860
      "Output - Loop 14" <- w864
    }
  }
